vi "ngi data packet JBV.vi"(0 "Dust Data Notifications":T9, 5 "list only event > 0":bool, 9 "mac adresses":T3, 12 "use correction":bool=TRUE) -> (1 "output waveforms":cluster{waveform(dbl)[], waveform(dbl)[]}, 2 "NGI  packets dust":cluster{"MAc Adress":string, "data":string}[](array[cluster]), 3 "Adjustable Parameters":T4(array[cluster]) {"ACMP0 ch" items=["Geophone 1"=0, "Geophone 2"=3, "Geophone 3"=4, "Geophone 4"=5]; "ACMP1 ch" items=["Geophone 2"=1, "Geophone 3"=2, "Geophone 4"=3]}, 6 "Avalanch JBV":T1(array[cluster]) {"A2 mean" format="%.1f"; "A1 mean" format="%.1f"; "A1 std" format="%.1f"; "A2 std" format="%.1f"}, 8 "Recent events":T5(array[cluster]) {"SPS" format="%.1f"}, 10 "Is Logging":T7(array[cluster]), 11 "AUX data":T2(array[cluster]) {"Node configuration"."configuration" items=[""=100, "Radio Repeater"=0, "Geofon"=1, "Sensornode"=2, "Infralyd"=4, "Jernbane"=3]; "Node configuration"."radio config" items=[""=100, "Smartmesh IP"=0]; "batteri (V)" format="%.3g"; "temperatur (c)" format="%.1g"; "?" format="%#.5g"}, 13 "Downloaded dataset":T6(array[cluster]), 14 "last packet type":u8[](array[numeric]), 15 "Avalanch Packets":T8(array[cluster]) {"A1 std" format="%.1g"; "A2 std" format="%.1g"; "A3 std" format="%.1g"; "A4 std" format="%.1g"; "A1 rat" format="%.1g"; "A2 rat" format="%.1g"; "A3 rat" format="%.1g"; "A4 rat" format="%.1g"})   [LabVIEW 2017]
panel:
  out "data":string
  out "sps":dbl
  out "num_samples":u16
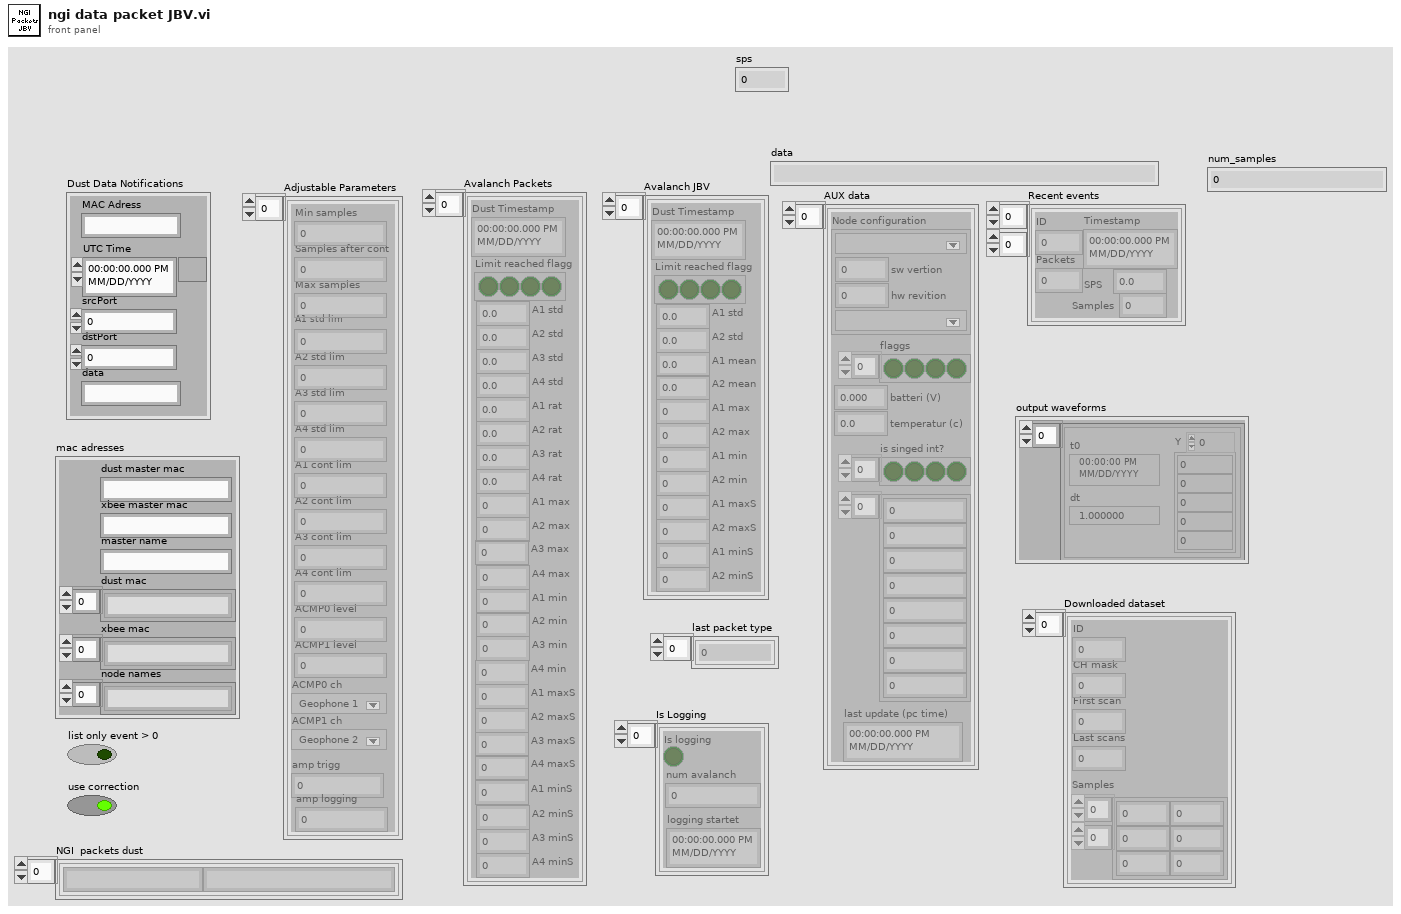
[diagram p1: front panel]
types:
  T1 = cluster{"Dust Timestamp":timestamp, "Limit reached flagg":bool[], "A1 std":sgl, "A2 std":sgl, "A1 mean":sgl, "A2 mean":sgl, "A1 max":i32, "A2 max":i32, "A1 min":i32, "A2 min":i32, "A1 maxS":u16, "A2 maxS":u16, "A1 minS":u16, "A2 minS":u16}[]
  T2 = cluster{"Node configuration":cluster{"configuration":u8, "sw vertion":u8, "hw revition":u8, "radio config":u8}, "flaggs":bool[], "batteri (V)":dbl, "temperatur (c)":dbl, "is singed int?":bool[], dbl[], "last update (pc time)":timestamp}[]
  T3 = cluster{"dust master mac":string, "xbee master mac":string, "master name":string, "dust mac":string[], "xbee mac":string[], "node names":string[]}
  T4 = cluster{"Min samples":u32, "Samples after cont":u32, "Max samples":u32, "A1 std lim":sgl, "A2 std lim":sgl, "A3 std lim":sgl, "A4 std lim":sgl, "A1 cont lim":sgl, "A2 cont lim":sgl, "A3 cont lim":sgl, "A4 cont lim":sgl, "ACMP0 level":u32, "ACMP1 level":u32, "ACMP0 ch":u8, "ACMP1 ch":u8, "amp trigg":u16, "amp logging":u16}[]
  T5 = cluster{"ID":u16, "Timestamp":timestamp, "Packets":u16, "SPS":dbl, "Samples":u16}[][]
  T6 = cluster{"ID":u16, "CH mask":u8, "First scan":u32, "Last scans":u32, "Samples":i32[][]}[]
  T7 = cluster{"Is logging":bool, "num avalanch":u16, "logging startet":timestamp}[]
  T8 = cluster{"Dust Timestamp":timestamp, "Limit reached flagg":bool[], "A1 std":sgl, "A2 std":sgl, "A3 std":sgl, "A4 std":sgl, "A1 rat":sgl, "A2 rat":sgl, "A3 rat":sgl, "A4 rat":sgl, "A1 max":u16, "A2 max":u16, "A3 max":u16, "A4 max":u16, "A1 min":u16, "A2 min":u16, "A3 min":u16, "A4 min":u16, "A1 maxS":u16, "A2 maxS":u16, "A3 maxS":u16, "A4 maxS":u16, "A1 minS":u16, "A2 minS":u16, "A3 minS":u16, "A4 minS":u16}[]
  T9 = cluster{"MAC Adress":string, "UTC Time":timestamp, "srcPort":u16, "dstPort":u16, "data":string}
  T10 = cluster{"Dust Timestamp":timestamp, "Boolean array":bool[], "default value 1":sgl, "default value 1":sgl, "default value 1":sgl, "default value 1":sgl, "default value 1":i32, "default value 1":i32, "default value 1":i32, "default value 1":i32, "default value 1":u16, "default value 1":u16, "default value 1":u16, "default value 1":u16}
  T11 = cluster{cluster{"configuration":i32, "sw vertion":u8, "hw revition":u8, "radio config":i32}, "flaggs":bool[], "batteri (V)":dbl, "temperatur (c)":dbl, "singed int":bool[], dbl[], "last update (pc time)":timestamp}
  T12 = cluster{"Dust Timestamp":timestamp, "Boolean array":bool[], "default value 1":sgl, "default value 1":sgl, "default value 1":sgl, "default value 1":sgl, "default value 1":sgl, "default value 1":sgl, "default value 1":sgl, "default value 1":sgl, "default value 1":u16, "default value 1":u16, "default value 1":u16, "default value 1":u16, "default value 1":u16, "default value 1":u16, "default value 1":u16, "default value 1":u16, "default value 1":u16, "default value 1":u16, "default value 1":u16, "default value 1":u16, "default value 2":u16, "default value 3":u16, "default value 4":u16, "default value 5":u16}
  T13 = cluster{"ID":u16, "Timestamp":timestamp, "Num Packets":u16, "SPS":dbl, "Num samples":u16}
  T14 = cluster{bool, "default value 1":u16, "seconds since 1Jan1904":timestamp}
  T15 = cluster{"default value 1":u16, "default value 1":u8, "default value 1":u32, "default value 1":u32, i32[][]}
  T16 = cluster{"default value 1":u32, "default value 1":u32, "default value 1":u32, "default value 1":sgl, "default value 1":sgl, "default value 1":sgl, "default value 1":sgl, "default value 1":sgl, "default value 1":sgl, "default value 1":sgl, "default value 1":sgl, "default value 1":u32, "default value 1":u32, "default value 1":u8, "default value 1":u8, "default value 2":u16, "default value 3":u16}
  T17 = cluster{"ID":u16, "Timestamp":timestamp, "Num":u16, "Rødt lys":dbl, "Num 2":i32}
  T18 = enum16{"big-endian, network order", "native, host order", "little-endian"}
  T19 = cluster{"Dust Timestamp":timestamp, "Boolean array":bool[], "default value 1":sgl, "default value 1":sgl, "default value 1":sgl, "default value 1":sgl, "default value 1":sgl, "default value 1":sgl, "default value 1":sgl, "default value 1":sgl, "default value 1":u16, "default value 1":u16, "default value 1":u16, "default value 1":u16, "default value 1":u16, "default value 1":u16, "default value 1":u16, "default value 1":u16, "default value 1":u16, "default value 1":u16, "default value 1":u16, "default value 1":u16, "default value 2":u16, "default value 3":u16, "default value 4":u16, "default value 5":u16}[]
  T20 = cluster{cluster{"configuration":i32, "sw vertion":u8, "hw revition":u8, "radio config":i32}, "flaggs":bool[], "batteri (V)":dbl, "temperatur (c)":dbl, "singed int":bool[], dbl[], "last update (pc time)":timestamp}[]
  T21 = cluster{"Dust Timestamp":timestamp, "Boolean array":bool[], "default value 1":sgl, "default value 1":sgl, "default value 1":sgl, "default value 1":sgl, "default value 1":i32, "default value 1":i32, "default value 1":i32, "default value 1":i32, "default value 1":u16, "default value 1":u16, "default value 1":u16, "default value 1":u16}[]
  T22 = cluster{"ID":u16, "Timestamp":timestamp, "Num Packets":u16, "SPS":dbl, "Num samples":u16}[][]
  T23 = cluster{"default value 1":u32, "default value 1":u32, "default value 1":u32, "default value 1":sgl, "default value 1":sgl, "default value 1":sgl, "default value 1":sgl, "default value 1":sgl, "default value 1":sgl, "default value 1":sgl, "default value 1":sgl, "default value 1":u32, "default value 1":u32, "default value 1":u8, "default value 1":u8, "default value 2":u16, "default value 3":u16}[]
  T24 = cluster{bool, "default value 1":u16, "seconds since 1Jan1904":timestamp}[]
  T25 = cluster{"default value 1":u16, "default value 1":u8, "default value 1":u32, "default value 1":u32, i32[][]}[]
  T26 = cluster{"Dust Timestamp":timestamp, "Boolean array":bool[], "default value 1":sgl, "default value 1":sgl, "default value 1":sgl, "default value 1":sgl, sgl, sgl, sgl, sgl, "default value 1":u16, "default value 1":u16, "default value 1":u16, "default value 1":u16, "default value 1":u16, "default value 1":u16, "default value 1":u16, "default value 1":u16, "default value 1":u16, "default value 1":u16, "default value 1":u16, "default value 1":u16, "default value 1":u16, "default value 1":u16, "default value 1":u16, "default value 1":u16}
  T27 = cluster{"Dust Timestamp":timestamp, "Boolean array":bool[], "default value 1":sgl, "default value 1":sgl, "default value 1":sgl, "default value 1":sgl, i32, i32, i32, i32, "default value 1":u16, "default value 1":u16, "default value 1":u16, "default value 1":u16}
  T28 = cluster{"Dust Timestamp":timestamp, "Boolean array":bool[], "default value 1":sgl, "default value 1":sgl, "default value 1":sgl, "default value 1":sgl, i32, "default value 1":i32, i32, "default value 1":i32, "default value 1":u16, "default value 1":u16, "default value 1":u16, "default value 1":u16}
  T29 = cluster{"default value 1":u16, "Dust Timestamp":timestamp, "default value 1":u16, dbl, "default value 1":u16}
  T30 = cluster{"ID":u16, "Timestamp":timestamp, "Num Packets":u16, "SPS":dbl, "Num 2":i32}[]
  T31 = cluster{"default value 1":u32, "default value 1":u32, "default value 1":u32, "default value 1":sgl, "default value 1":sgl, "default value 1":sgl, "default value 1":sgl, "default value 1":sgl, "default value 1":sgl, "default value 1":sgl, "default value 1":sgl, u32, u32, "default value 1":u8, "default value 1":u8, "default value 1":u16, "default value 1":u16}
  T32 = cluster{cluster{u8, u8, u8, u8}, "Boolean array":bool[], dbl, dbl, "Boolean array":bool[], dbl[], "seconds since 1Jan1904":timestamp}
  T33 = cluster{"ID":u16, "Timestamp":timestamp, "Num Packets":u16, "SPS":dbl, "Num 2":i32}[][]
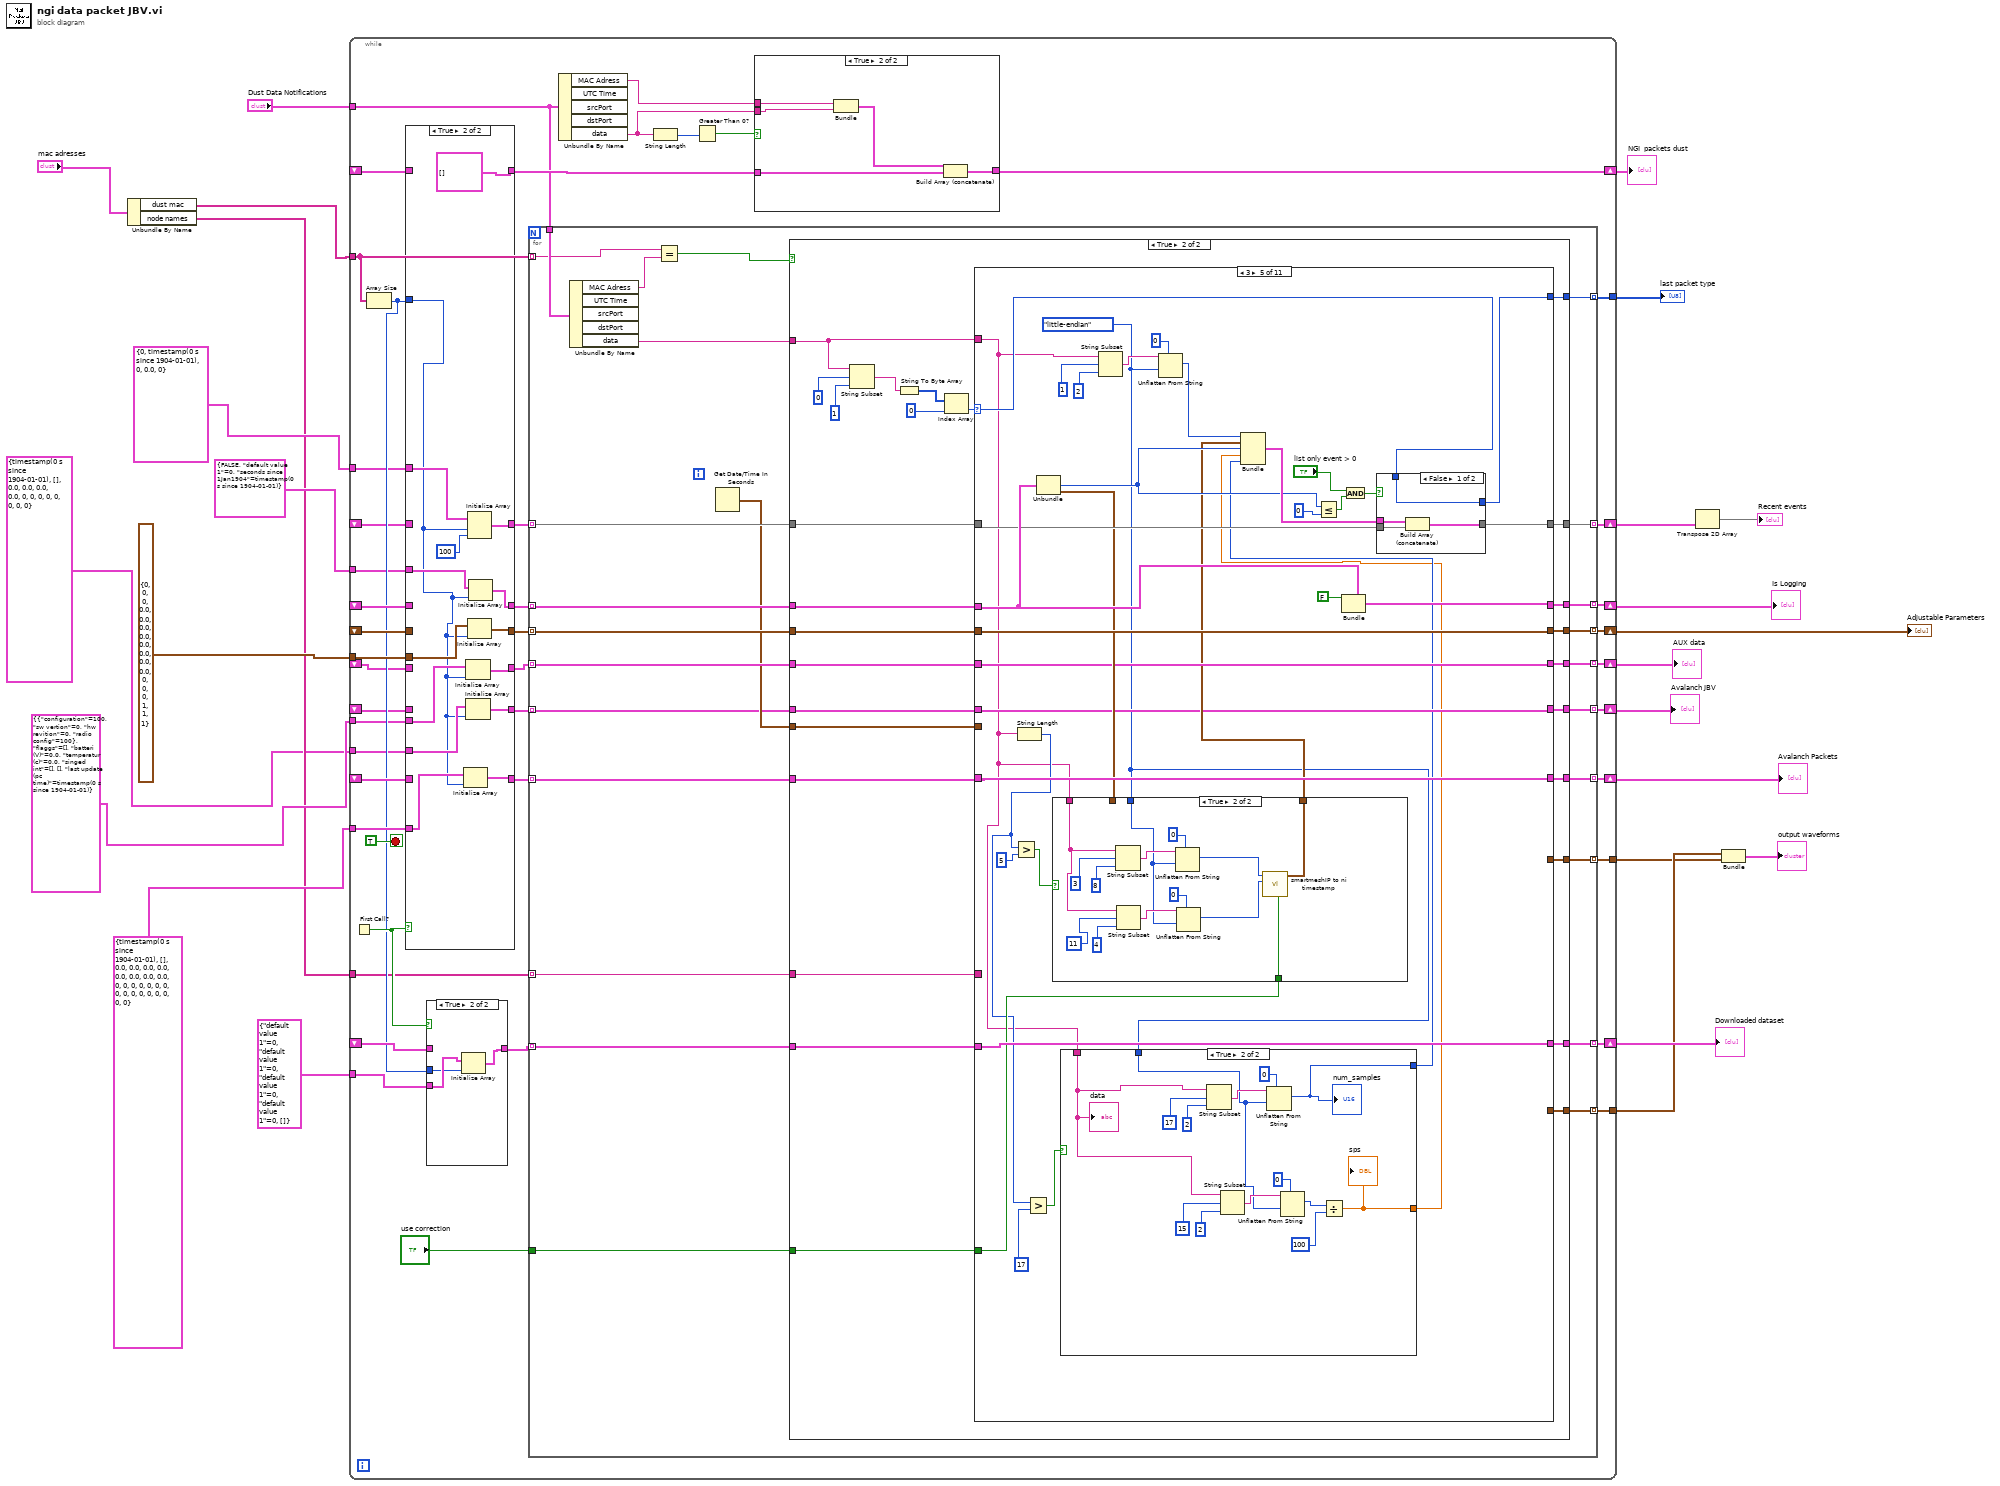
[diagram p0: block diagram]
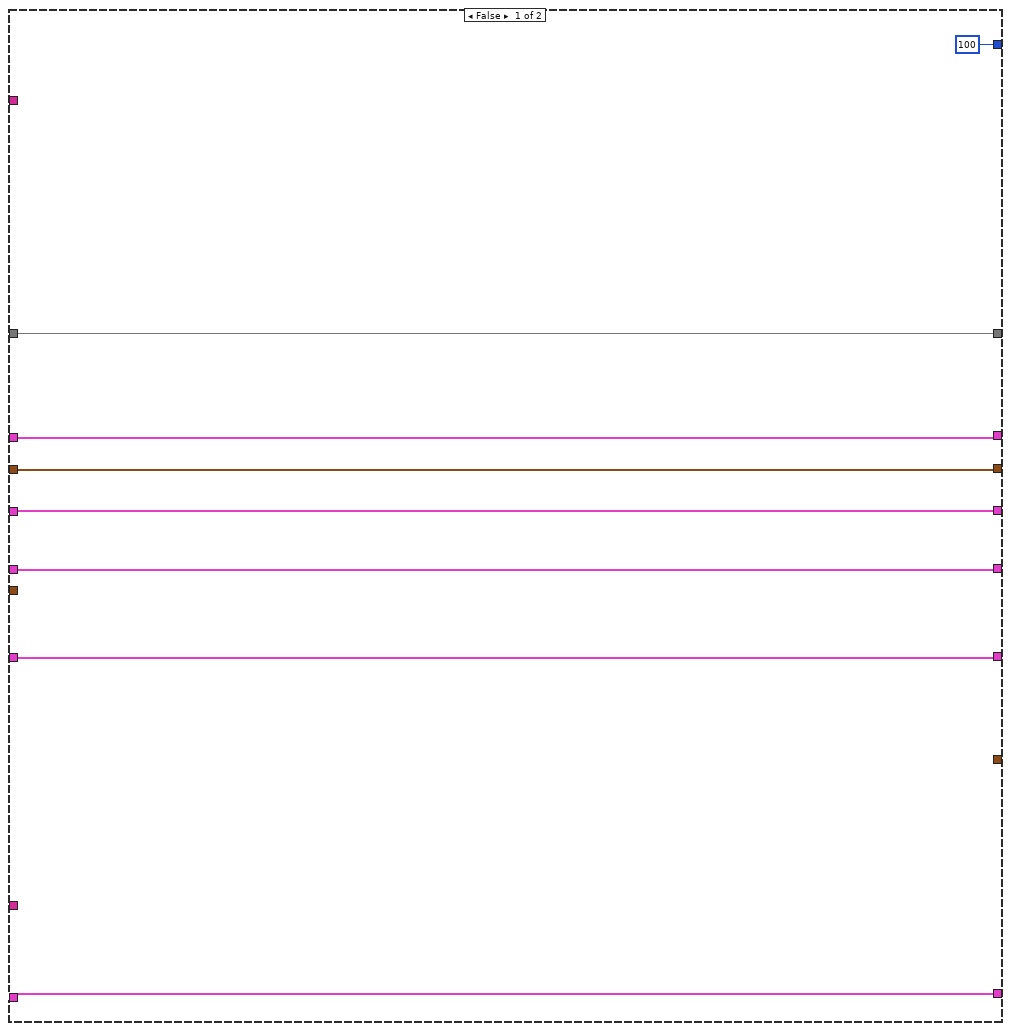
[diagram p3: hidden frame]
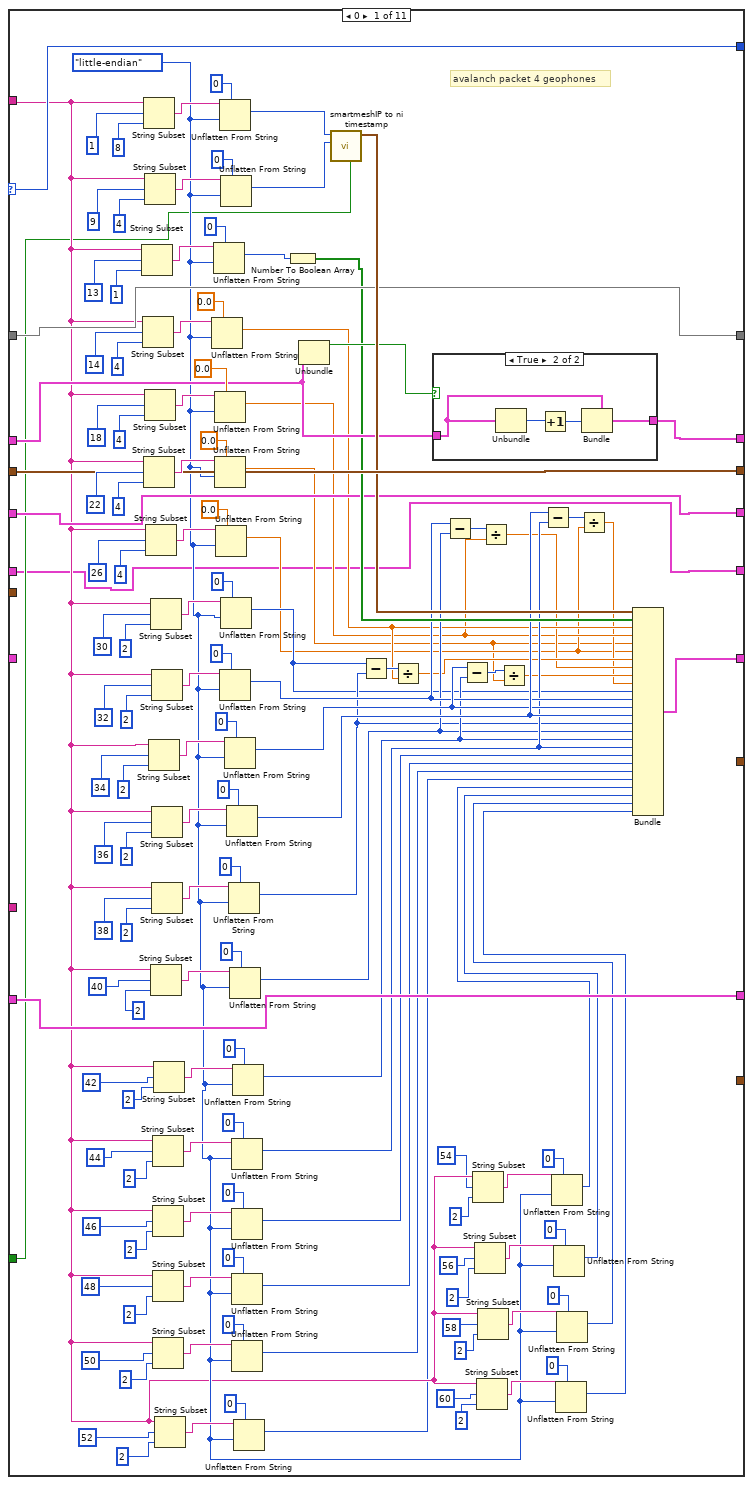
[diagram p4: hidden frame]
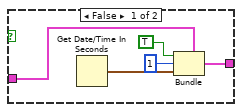
[diagram p5: hidden frame]
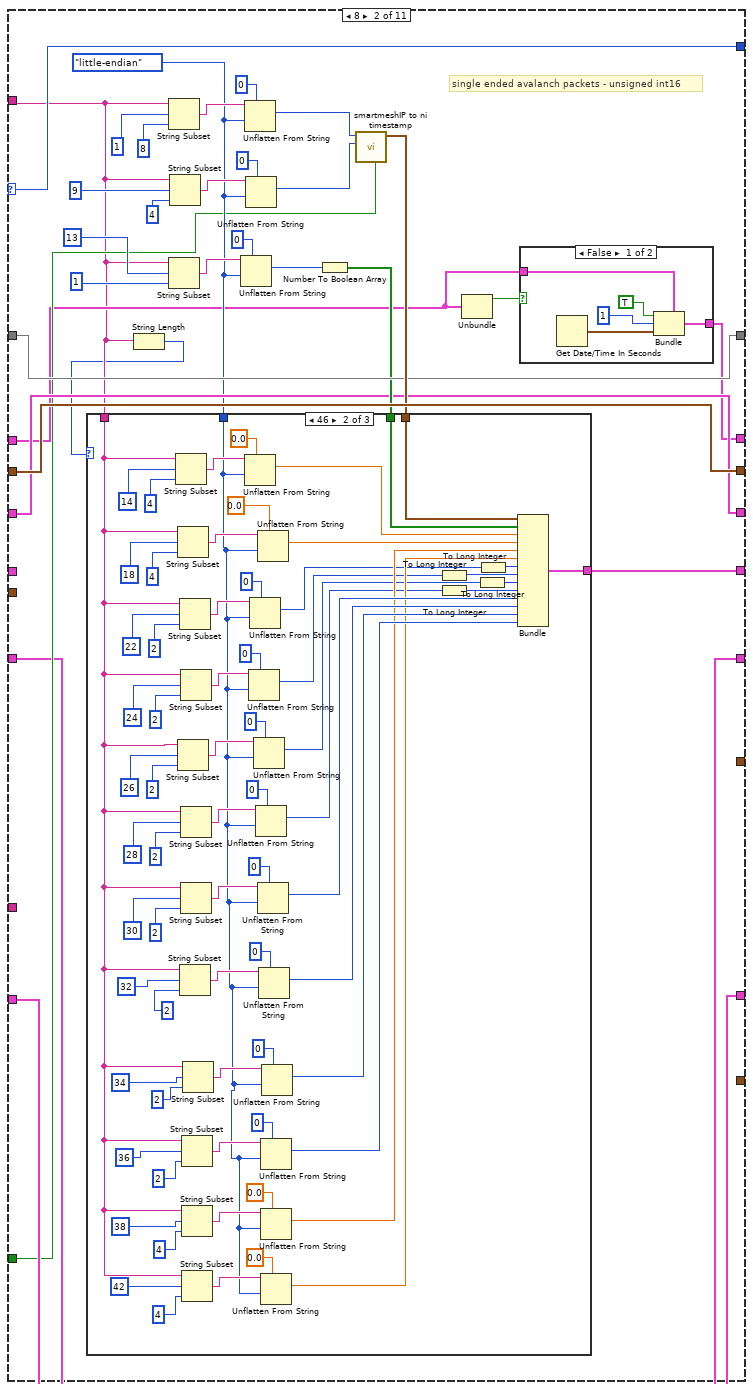
[diagram p6: hidden frame]
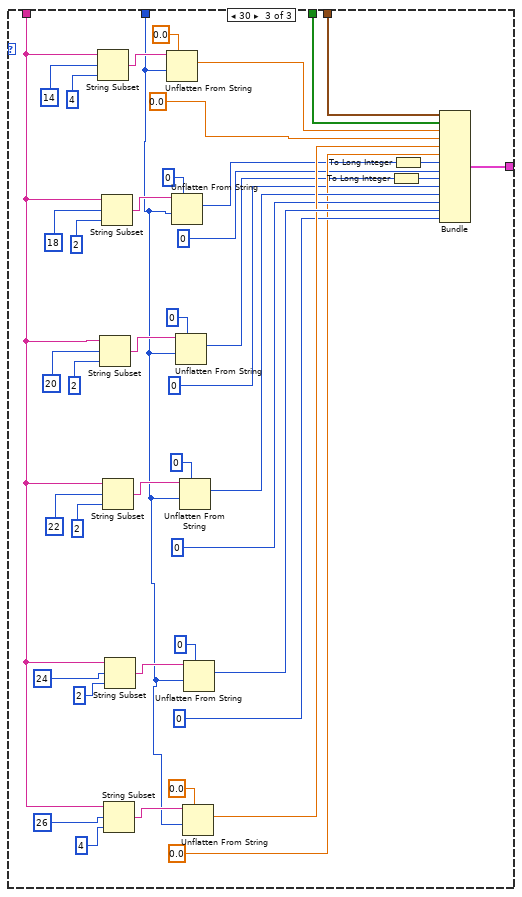
[diagram p8: hidden frame]
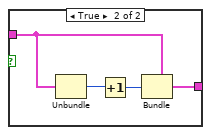
[diagram p9: hidden frame]
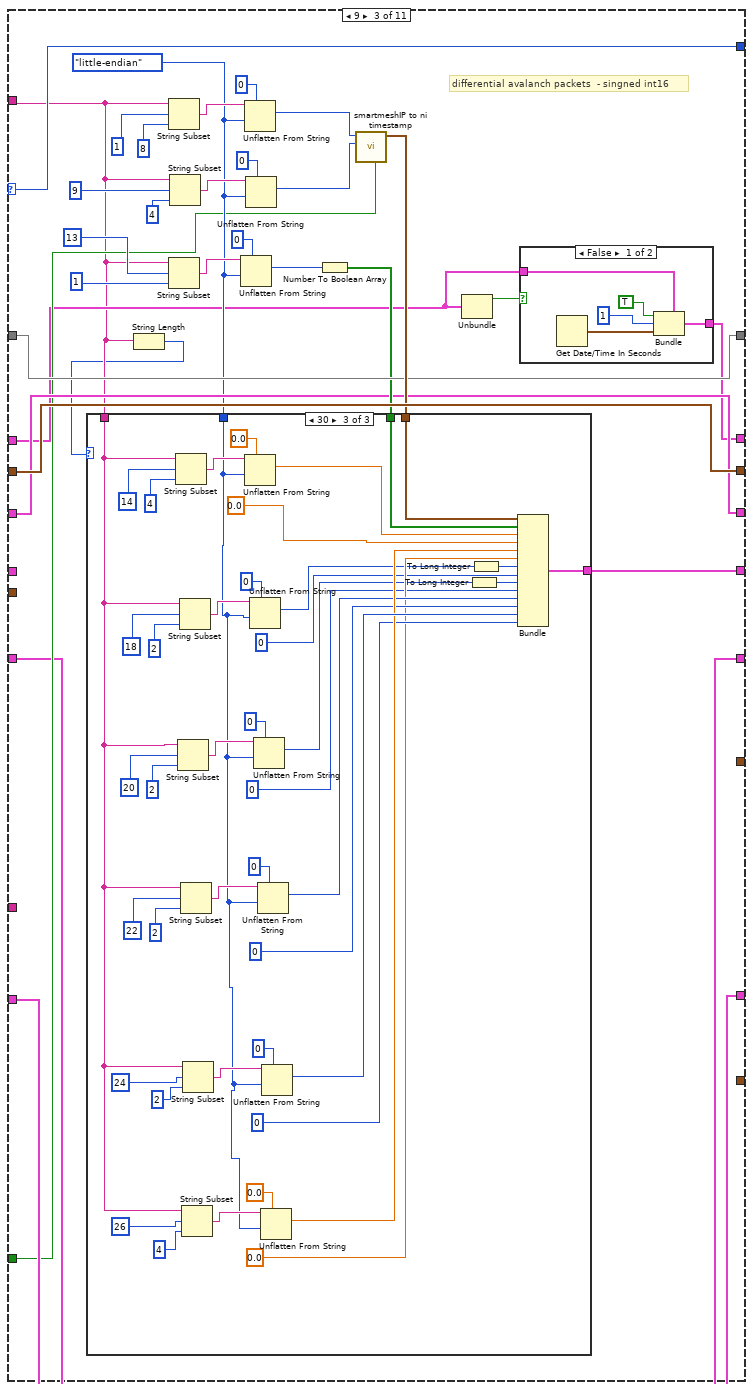
[diagram p10: hidden frame]
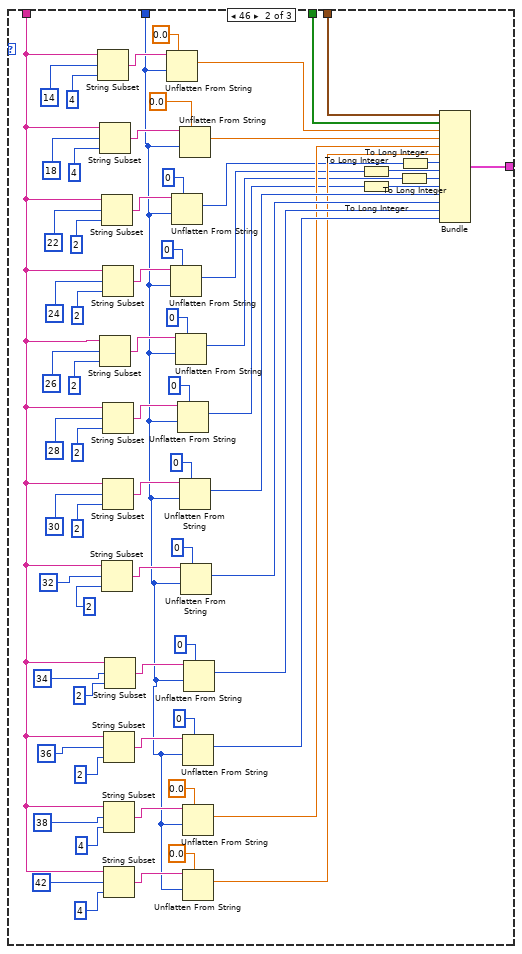
[diagram p12: hidden frame]
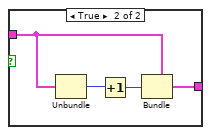
[diagram p13: hidden frame]
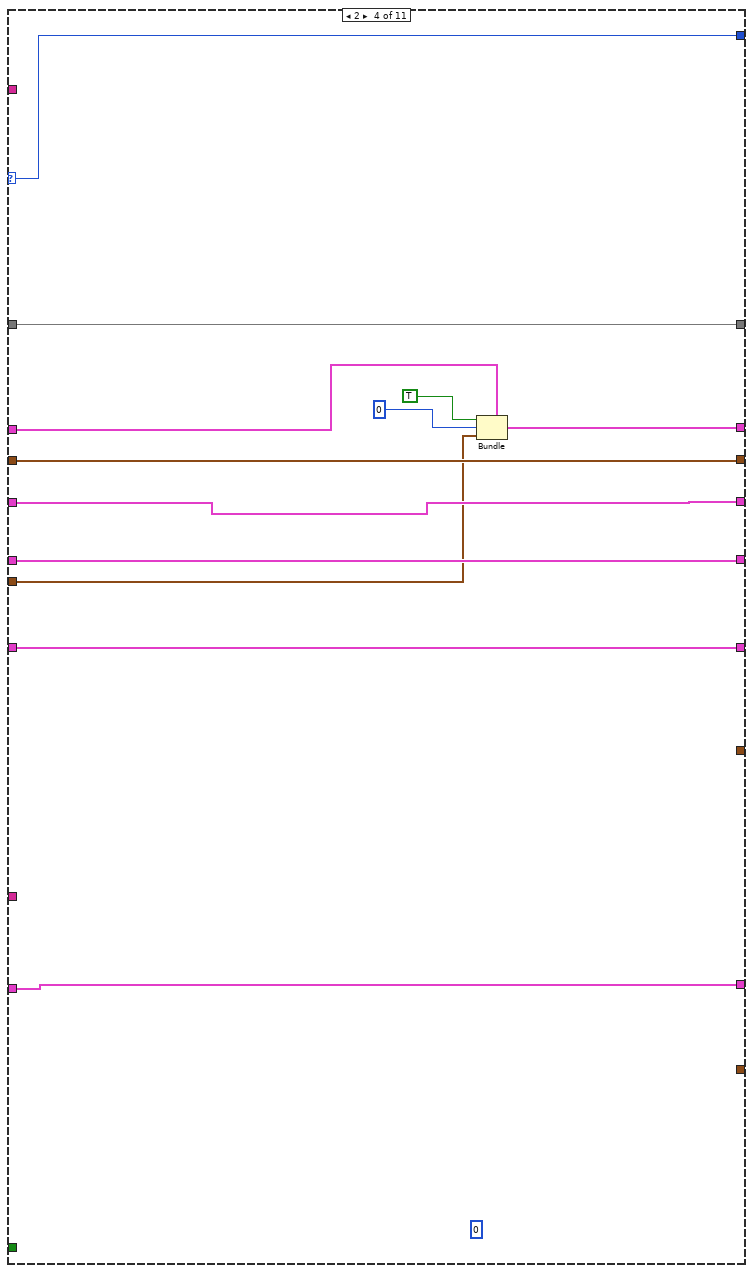
[diagram p14: hidden frame]
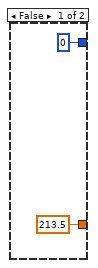
[diagram p15: hidden frame]
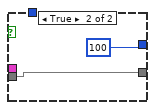
[diagram p16: hidden frame]
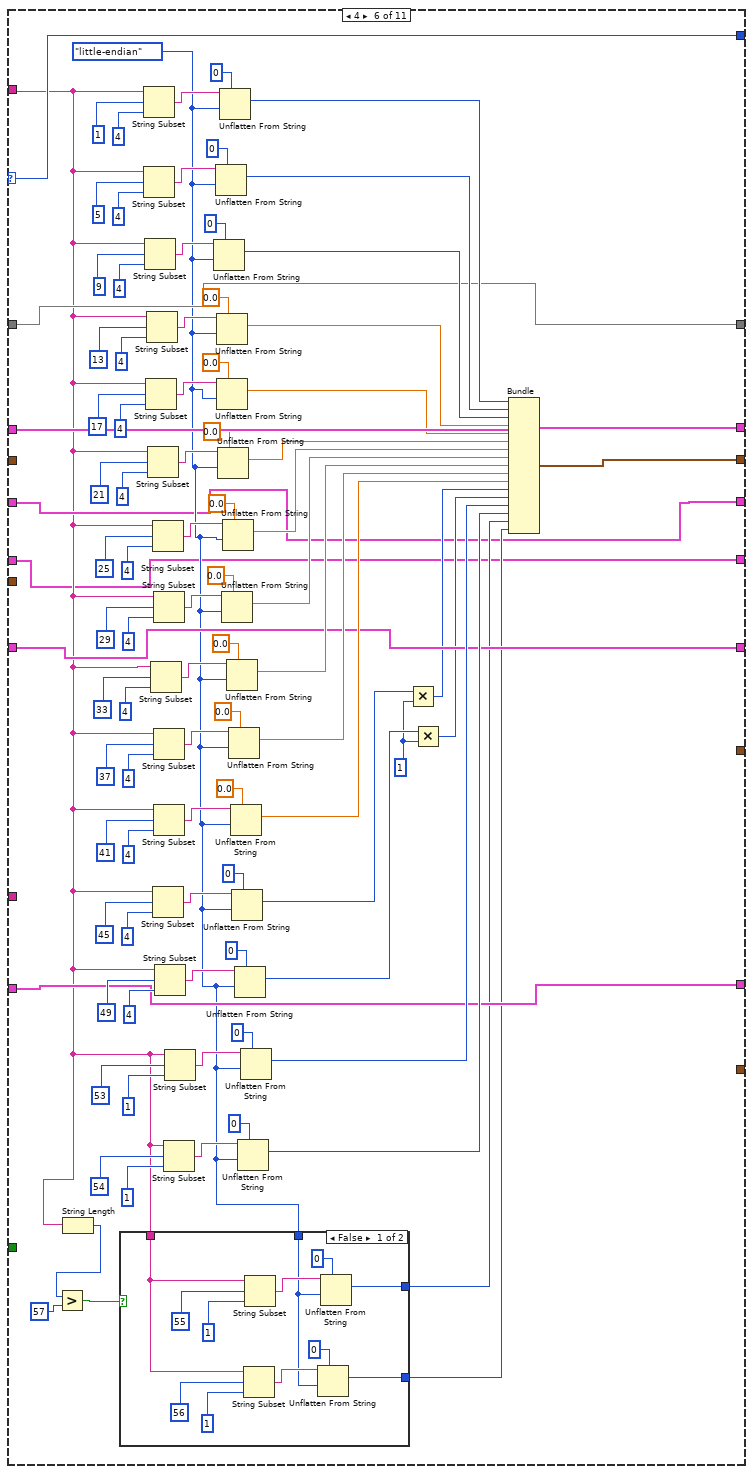
[diagram p18: hidden frame]
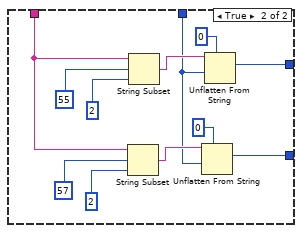
[diagram p19: hidden frame]
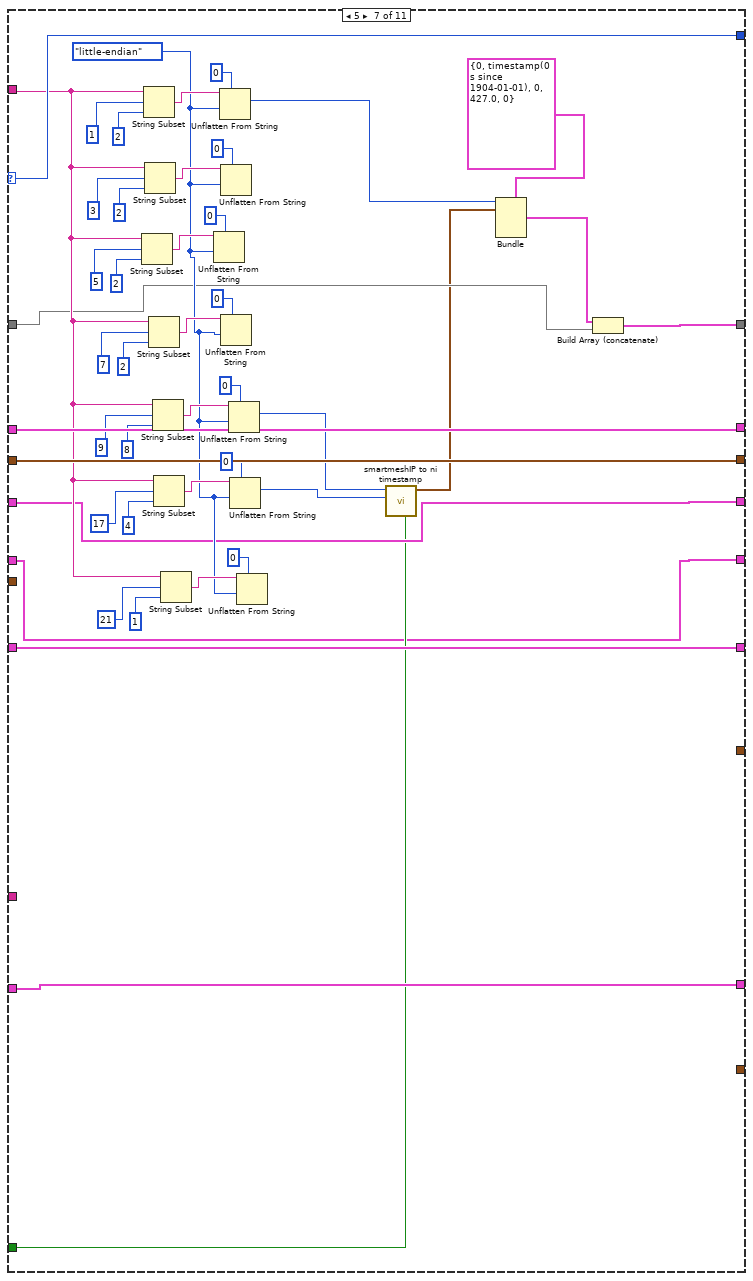
[diagram p20: hidden frame]
diagram:
  n1 = Unbundle By Name("mac adresses") -> ("dust mac"=w11:string[], "node names"=w3:string[])
  n2 = while {
    tunnel: "Dust Data Notifications" -> [w61]
    tunnel: w11 -> [w60]
    shift-right: [w64] -> w23
    shift-left: _ -> [w62]
    shift-right: [w59] -> w17
    shift-left: _ -> [w57]
    shift-right: [w56] -> w12
    shift-left: _ -> [w55]
    tunnel: T16 {"default value 1"=0, "default value 1"=0, "default value 1"=0, "default value 1"=0.0, "default value 1"=0.0, "default value 1"=0.0, "default value 1"=0.0, "default value 1"=0.0, "default value 1"=0.0, "default value 1"=0.0, "default value 1"=0.0, "default value 1"=0, "default value 1"=0, "default value 1"=0, "default value 1"=1, "default value 2"=1, "default value 3"=1} -> [w53]
    tunnel: [w52] -> w21
    shift-right: [w51] -> w19
    shift-left: _ -> [w49]
    tunnel: T12 {"Dust Timestamp"=timestamp(0 s since 1904-01-01), "Boolean array"=[], "default value 1"=0.0, "default value 1"=0.0, "default value 1"=0.0, "default value 1"=0.0, "default value 1"=0.0, "default value 1"=0.0, "default value 1"=0.0, "default value 1"=0.0, "default value 1"=0, "default value 1"=0, "default value 1"=0, "default value 1"=0, "default value 1"=0, "default value 1"=0, "default value 1"=0, "default value 1"=0, "default value 1"=0, "default value 1"=0, "default value 1"=0, "default value 1"=0, "default value 2"=0, "default value 3"=0, "default value 4"=0, "default value 5"=0} -> [w48]
    shift-right: [w47] -> w16
    shift-left: _ -> [w45]
    tunnel: T15 {"default value 1"=0, "default value 1"=0, "default value 1"=0, "default value 1"=0, []} -> [w44]
    shift-right: [w38] -> w14
    shift-left: _ -> [w37]
    tunnel: T14 {FALSE, "default value 1"=0, "seconds since 1Jan1904"=timestamp(0 s since 1904-01-01)} -> [w40]
    tunnel: T13 {"ID"=0, "Timestamp"=timestamp(0 s since 1904-01-01), "Num Packets"=0, "SPS"=0.0, "Num samples"=0} -> [w39]
    tunnel: [w36] -> w5
    tunnel: w3 -> [w35]
    tunnel: [w34] -> w6
    shift-right: [w33] -> w8
    shift-left: _ -> [w31]
    tunnel: T11 {{"configuration"=100, "sw vertion"=0, "hw revition"=0, "radio config"=100}, "flaggs"=[], "batteri (V)"=0.0, "temperatur (c)"=0.0, "singed int"=[], [], "last update (pc time)"=timestamp(0 s since 1904-01-01)} -> [w30]
    shift-right: [w28] -> w2
    shift-left: _ -> [w27]
    tunnel: T10 {"Dust Timestamp"=timestamp(0 s since 1904-01-01), "Boolean array"=[], "default value 1"=0.0, "default value 1"=0.0, "default value 1"=0.0, "default value 1"=0.0, "default value 1"=0, "default value 1"=0, "default value 1"=0, "default value 1"=0, "default value 1"=0, "default value 1"=0, "default value 1"=0, "default value 1"=0} -> [w25]
    stop <- TRUE stop-if-true
    n3 = First Call?() -> (First Call?: T/F=w42:bool)
    n4 = Array Size(array=w60) -> (size(s)=w41:i32)
    n5 = case shown="True" w42 {
      tunnel: [w1077 cluster{"MAc Adress":string, "data":string}[] []] -> w63
      tunnel: w62 -> [w1077 _]
      tunnel: w41 -> [_ w1079]
      tunnel: [w1076 w1085] -> w58
      tunnel: w57 -> [w1076 _]
      tunnel: [w1075 w1091] -> w54
      tunnel: w55 -> [w1075 _]
      tunnel: w53 -> [_ w1092]
      tunnel: [w1074 w1090] -> w50
      tunnel: w49 -> [w1074 _]
      tunnel: w48 -> [_ w1089]
      tunnel: [w1073 w1083] -> w43
      tunnel: w37 -> [w1073 _]
      tunnel: w40 -> [_ w1086]
      tunnel: w39 -> [_ w1084]
      tunnel: [w1072 w1081] -> w32
      tunnel: w31 -> [w1072 _]
      tunnel: w30 -> [_ w1082]
      tunnel: w27 -> [w1071 _]
      tunnel: [w1071 w1078] -> w26
      tunnel: w25 -> [_ w1080]
      frame False {
      }
      frame True {
        n6 = Initialize Array(w1089, w1079) -> (w1090:T19)
        n7 = Initialize Array(w1082, w1079) -> (w1081:T20)
        n8 = Initialize Array(w1080, w1079) -> (w1078:T21)
        n9 = Initialize Array(w1084, w1079, 100 ("dimension size")) -> (w1083:T22)
        n10 = Initialize Array(w1092, w1079) -> (w1091:T23)
        n11 = Initialize Array(w1086, w1079) -> (w1085:T24)
      }
    }
    n12 = case shown="True" w42 {
      tunnel: [w70 w71] -> w46
      tunnel: w45 -> [w70 _]
      tunnel: w44 -> [_ w73]
      tunnel: w41 -> [_ w72]
      frame False {
      }
      frame True {
        n13 = Initialize Array(w73, w72) -> (w71:T25)
      }
    }
    n14 = for {
      tunnel: w60 -> [w97] mode=indexing
      tunnel: w61 -> [w98]
      tunnel: [w96] -> w59 mode=indexing
      tunnel: w58 -> [w95] mode=indexing
      tunnel: [w94] -> w56 mode=indexing
      tunnel: w54 -> [w93] mode=indexing
      tunnel: [w92] -> w52 mode=indexing
      tunnel: [w91] -> w51 mode=indexing
      tunnel: w50 -> [w90] mode=indexing
      tunnel: [w89] -> w47 mode=indexing
      tunnel: w46 -> [w88] mode=indexing
      tunnel: [w87] -> w38 mode=indexing
      tunnel: w43 -> [w86] mode=indexing
      tunnel: [w85] -> w36 mode=indexing
      tunnel: w35 -> [w84] mode=indexing
      tunnel: [w83] -> w34 mode=indexing
      tunnel: [w82] -> w33 mode=indexing
      tunnel: w32 -> [w81] mode=indexing
      tunnel: "use correction" -> [w79]
      tunnel: [w75] -> w28 mode=indexing
      tunnel: w26 -> [w74] mode=indexing
      n15 = Unbundle By Name(w98) -> ("MAC Adress"=w80:string, "data"=w76:string)  [unwired: 3 out]
      n16 = Equal?(x=w97, y=w80) -> (x = y?=w77:bool)
      n17 = Get Date/Time In Seconds() -> (seconds since 1Jan1904=w78:timestamp)
      n18 = case shown="True" w77 {
        tunnel: w76 -> [_ w121]
        tunnel: [w106 w132] -> w96
        tunnel: w95 -> [w106 w133]
        tunnel: [w105 w131] -> w94
        tunnel: w93 -> [w105 w130]
        tunnel: [u8 100 w129] -> w92
        tunnel: [w104 w128] -> w91
        tunnel: w90 -> [w104 w127]
        tunnel: [w103 w119] -> w89
        tunnel: w88 -> [w103 w118]
        tunnel: w78 -> [_ w117]
        tunnel: [w102 w116] -> w87
        tunnel: w86 -> [w102 w115]
        tunnel: [_ w114] -> w85
        tunnel: w84 -> [_ w113]
        tunnel: [_ w112] -> w83
        tunnel: [w100 w111] -> w82
        tunnel: w81 -> [w100 w110]
        tunnel: w79 -> [_ w109]
        tunnel: [w99 w108] -> w75
        tunnel: w74 -> [w99 w107]
        frame False {
        }
        frame True {
          n19 = String Subset(string=w121, offset (0)=0, length (rest)=1 ("length (rest)")) -> (substring=w126:string)
          n20 = String To Byte Array(string=w126) -> (unsigned byte array=w125:u8[])
          n21 = Index Array(array=w125, index=0) -> (element=w120:u8)
          n22 = case shown="3" w120 {
            selector: w120 -> [w226 w303 w455 w595 w611 w686 w823 w864 w920 w1015 _]
            tunnel: w133 -> [w210 w285 w437 w591 w621 w758 w817 w857 w913 w1009 w1070]
            tunnel: [w209 w283 w435 w590 w623 w758 w817 w857 w913 w1009 w1070] -> w132
            tunnel: w121 -> [w174 w282 w434 _ w597 w673 w800 w846 w902 w948 _]
            tunnel: [w225 w302 w454 w596 w631 w730 w818 w858 w914 w1010 w1069] -> w131
            tunnel: w130 -> [w225 w302 w454 w596 w631 _ w818 w858 w914 w1010 w1069]
            tunnel: [w226 w303 w455 w595 w610 w686 w823 w864 w920 w1015 u8 100] -> w129
            tunnel: [w223 w287 w439 w594 w630 w685 w816 w856 w912 w1008 w1068] -> w128
            tunnel: w127 -> [_ w287 w439 w594 w630 w685 w816 w856 w912 w1008 w1068]
            tunnel: [w216 w297 w449 w593 w629 w684 w797 w842 w898 w1007 w1067] -> w119
            tunnel: w118 -> [w216 w297 w449 w593 w629 w684 w797 _ _ w1007 w1067]
            tunnel: w117 -> [_ _ _ w585 _ _ _ _ _ w954 _]
            tunnel: [w212 w293 w445 w592 w624 w683 w793 w843 w899 w1006 w1066] -> w116
            tunnel: w115 -> [w212 w293 w445 w592 w620 w683 w794 w843 w899 w1006 w1066]
            tunnel: [_ _ _ _ _ _ _ _ _ w1002 _] -> w114
            tunnel: w113 -> [_ _ _ _ _ _ _ _ _ w996 _]
            tunnel: [_ _ _ _ _ _ _ _ _ w995 _] -> w112
            tunnel: [w206 w290 w442 w587 w615 w674 w788 w840 w896 w975 w1064] -> w111
            tunnel: w110 -> [w206 w290 w442 w587 w615 w674 w788 w840 w896 _ w1064]
            tunnel: w109 -> [w135 w288 w440 _ w604 _ w787 _ _ _ _]
            tunnel: [w134 w286 w438 w586 w605 w669 w786 w832 w888 w944 w1063] -> w108
            tunnel: w107 -> [w134 _ _ w586 w605 w669 w786 w832 w888 w944 w1063]
            frame 0 {
              w185 = T18."little-endian" ("byte order (0:big-endian, network order)")
              # "avalanch packet 4 geophones"
              n23 = String Subset(string=w174, offset (0)=13, length (rest)=1 ("length (rest)")) -> (substring=w236:string)
              n24 = String Subset(string=w174, offset (0)=14, length (rest)=4 ("length (rest)")) -> (substring=w235:string)
              n25 = String Subset(string=w174, offset (0)=1, length (rest)=8 ("length (rest)")) -> (substring=w249:string)
              n26 = String Subset(string=w174, offset (0)=22, length (rest)=4 ("length (rest)")) -> (substring=w233:string)
              n27 = String Subset(string=w174, offset (0)=9, length (rest)=4 ("length (rest)")) -> (substring=w219:string)
              n28 = String Subset(string=w174, offset (0)=18, length (rest)=4 ("length (rest)")) -> (substring=w234:string)
              n29 = String Subset(string=w174, offset (0)=26, length (rest)=4 ("length (rest)")) -> (substring=w232:string)
              n30 = String Subset(string=w174, offset (0)=34, length (rest)=2 ("length (rest)")) -> (substring=w229:string)
              n31 = String Subset(string=w174, offset (0)=30, length (rest)=2 ("length (rest)")) -> (substring=w231:string)
              n32 = String Subset(string=w174, offset (0)=40, length (rest)=2 ("length (rest)")) -> (substring=w222:string)
              n33 = String Subset(string=w174, offset (0)=32, length (rest)=2 ("length (rest)")) -> (substring=w230:string)
              n34 = String Subset(string=w174, offset (0)=36, length (rest)=2 ("length (rest)")) -> (substring=w228:string)
              n35 = String Subset(string=w174, offset (0)=38, length (rest)=2 ("length (rest)")) -> (substring=w227:string)
              n36 = String Subset(string=w174, offset (0)=44, length (rest)=2 ("length (rest)")) -> (substring=w202:string)
              n37 = String Subset(string=w174, offset (0)=46, length (rest)=2 ("length (rest)")) -> (substring=w200:string)
              n38 = String Subset(string=w174, offset (0)=48, length (rest)=2 ("length (rest)")) -> (substring=w198:string)
              n39 = String Subset(string=w174, offset (0)=50, length (rest)=2 ("length (rest)")) -> (substring=w196:string)
              n40 = String Subset(string=w174, offset (0)=42, length (rest)=2 ("length (rest)")) -> (substring=w204:string)
              n41 = String Subset(string=w174, offset (0)=52, length (rest)=2 ("length (rest)")) -> (substring=w186:string)
              n42 = Unflatten From String(type=sgl 0.0 ("default value 1"), binary string=w235, byte order (0:big-endian, network order)=w185) -> (value=w145:sgl)  [unwired: 2 in, 2 out]
              n43 = Unflatten From String(type=u8 0 ("default value 1"), binary string=w236, byte order (0:big-endian, network order)=w185) -> (value=w208:u8)  [unwired: 2 in, 2 out]
              n44 = Unflatten From String(type=sgl 0.0 ("default value 1"), binary string=w234, byte order (0:big-endian, network order)=w185) -> (value=w142:sgl)  [unwired: 2 in, 2 out]
              n45 = Unflatten From String(type=sgl 0.0 ("default value 1"), binary string=w233, byte order (0:big-endian, network order)=w185) -> (value=w136:sgl)  [unwired: 2 in, 2 out]
              n46 = Unflatten From String(type=sgl 0.0 ("default value 1"), binary string=w232, byte order (0:big-endian, network order)=w185) -> (value=w137:sgl)  [unwired: 2 in, 2 out]
              n47 = Unflatten From String(type=i64 0 ("default value 1"), binary string=w249, byte order (0:big-endian, network order)=w185) -> (value=w215:i64)  [unwired: 2 in, 2 out]
              n48 = Unflatten From String(type=u16 0 ("default value 1"), binary string=w230, byte order (0:big-endian, network order)=w185) -> (value=w153:u16)  [unwired: 2 in, 2 out]
              n49 = Unflatten From String(type=0 ("default value 1"), binary string=w219, byte order (0:big-endian, network order)=w185) -> (value=w214:i32)  [unwired: 2 in, 2 out]
              n50 = Unflatten From String(type=u16 0 ("default value 1"), binary string=w231, byte order (0:big-endian, network order)=w185) -> (value=w147:u16)  [unwired: 2 in, 2 out]
              n51 = Unflatten From String(type=u16 0 ("default value 1"), binary string=w229, byte order (0:big-endian, network order)=w185) -> (value=w154:u16)  [unwired: 2 in, 2 out]
              n52 = Unflatten From String(type=u16 0 ("default value 1"), binary string=w228, byte order (0:big-endian, network order)=w185) -> (value=w155:u16)  [unwired: 2 in, 2 out]
              n53 = Unflatten From String(type=u16 0 ("default value 1"), binary string=w227, byte order (0:big-endian, network order)=w185) -> (value=w149:u16)  [unwired: 2 in, 2 out]
              n54 = Unflatten From String(type=u16 0 ("default value 1"), binary string=w222, byte order (0:big-endian, network order)=w185) -> (value=w150:u16)  [unwired: 2 in, 2 out]
              n55 = Unflatten From String(type=u16 0 ("default value 1"), binary string=w202, byte order (0:big-endian, network order)=w185) -> (value=w152:u16)  [unwired: 2 in, 2 out]
              n56 = Unflatten From String(type=u16 0 ("default value 1"), binary string=w200, byte order (0:big-endian, network order)=w185) -> (value=w156:u16)  [unwired: 2 in, 2 out]
              n57 = Unflatten From String(type=u16 0 ("default value 1"), binary string=w198, byte order (0:big-endian, network order)=w185) -> (value=w157:u16)  [unwired: 2 in, 2 out]
              n58 = Unflatten From String(type=u16 0 ("default value 1"), binary string=w196, byte order (0:big-endian, network order)=w185) -> (value=w158:u16)  [unwired: 2 in, 2 out]
              n59 = Unflatten From String(type=u16 0 ("default value 1"), binary string=w204, byte order (0:big-endian, network order)=w185) -> (value=w151:u16)  [unwired: 2 in, 2 out]
              n60 = Unflatten From String(type=u16 0 ("default value 1"), binary string=w186, byte order (0:big-endian, network order)=w185) -> (value=w159:u16)  [unwired: 2 in, 2 out]
              n61 = Number To Boolean Array(number=w208) -> (Boolean array=w207:bool[])
              n62 = Unbundle(w210) -> (w211:bool)  [unwired: 2 out]
              n63 = call "smartmeshIP to ni timestamp.vi"("use correction"=w135, "microeconds"=w214, "seconds"=w215) -> ("Dust Timestamp"=w213:timestamp)  [unwired: 8 in]
              n64 = Subtract(x=w147, y=w149) -> (x-y=w148:u16)
              n65 = Divide(x=w148, y=w145) -> (x/y=w146:sgl)
              n66 = case shown="True" w211 {
                tunnel: w210 -> [w276 w280]
                tunnel: [w273 w277] -> w209
                frame False {
                  n67 = Get Date/Time In Seconds() -> (seconds since 1Jan1904=w272:timestamp)
                  n68 = Bundle(cluster=w276, TRUE, "default value 1"=u16 1, "seconds since 1Jan1904"=w272) -> (w273:T14)
                }
                frame True {
                  n69 = Unbundle(w280) -> ("default value 1"=w278:u16)  [unwired: 2 out]
                  n70 = Increment(x=w278) -> (x+1=w279:u16)
                  n71 = Bundle(cluster=w280, "default value 1"=w279) -> (w277:T14)  [unwired: 2 in]
                }
              }
              n72 = Subtract(x=w153, y=w150) -> (x-y=w144:u16)
              n73 = Subtract(x=w154, y=w151) -> (x-y=w141:u16)
              n74 = String Subset(string=w174, offset (0)=54, length (rest)=2 ("length (rest)")) -> (substring=w194:string)
              n75 = String Subset(string=w174, offset (0)=56, length (rest)=2 ("length (rest)")) -> (substring=w192:string)
              n76 = String Subset(string=w174, offset (0)=60, length (rest)=2 ("length (rest)")) -> (substring=w188:string)
              n77 = String Subset(string=w174, offset (0)=58, length (rest)=2 ("length (rest)")) -> (substring=w190:string)
              n78 = Divide(x=w144, y=w142) -> (x/y=w143:sgl)
              n79 = Divide(x=w141, y=w136) -> (x/y=w140:sgl)
              n80 = Subtract(x=w155, y=w152) -> (x-y=w139:u16)
              n81 = Unflatten From String(type=u16 0 ("default value 1"), binary string=w194, byte order (0:big-endian, network order)=w185) -> (value=w160:u16)  [unwired: 2 in, 2 out]
              n82 = Unflatten From String(type=u16 0 ("default value 1"), binary string=w192, byte order (0:big-endian, network order)=w185) -> (value=w161:u16)  [unwired: 2 in, 2 out]
              n83 = Unflatten From String(type=u16 0 ("default value 1"), binary string=w188, byte order (0:big-endian, network order)=w185) -> (value=w163:u16)  [unwired: 2 in, 2 out]
              n84 = Unflatten From String(type=u16 0 ("default value 1"), binary string=w190, byte order (0:big-endian, network order)=w185) -> (value=w162:u16)  [unwired: 2 in, 2 out]
              n85 = Divide(x=w139, y=w137) -> (x/y=w138:sgl)
              n86 = Bundle("Dust Timestamp"=w213, "Boolean array"=w207, "default value 1"=w145, "default value 1"=w142, "default value 1"=w136, "default value 1"=w137, w146, w143, w140, w138, "default value 1"=w147, "default value 1"=w153, "default value 1"=w154, "default value 1"=w155, "default value 1"=w149, "default value 1"=w150, "default value 1"=w151, "default value 1"=w152, "default value 1"=w156, "default value 1"=w157, "default value 1"=w158, "default value 1"=w159, "default value 1"=w160, "default value 1"=w161, "default value 1"=w162, "default value 1"=w163) -> (w223:T26)  [unwired: 1 in]
            }
            frame 8 {
              w289 = T18."little-endian" ("byte order (0:big-endian, network order)")
              # "single ended avalanch packets - unsigned int16"
              n87 = String Length(string=w282) -> (length=w281:i32)
              n88 = String Subset(string=w282, offset (0)=1, length (rest)=8 ("length (rest)")) -> (substring=w307:string)
              n89 = String Subset(string=w282, offset (0)=13, length (rest)=1 ("length (rest)")) -> (substring=w304:string)
              n90 = String Subset(string=w282, offset (0)=9, length (rest)=4 ("length (rest)")) -> (substring=w299:string)
              n91 = Unflatten From String(type=u8 0 ("default value 1"), binary string=w304, byte order (0:big-endian, network order)=w289) -> (value=w292:u8)  [unwired: 2 in, 2 out]
              n92 = Unflatten From String(type=i64 0 ("default value 1"), binary string=w307, byte order (0:big-endian, network order)=w289) -> (value=w296:i64)  [unwired: 2 in, 2 out]
              n93 = Unflatten From String(type=0 ("default value 1"), binary string=w299, byte order (0:big-endian, network order)=w289) -> (value=w295:i32)  [unwired: 2 in, 2 out]
              n94 = Number To Boolean Array(number=w292) -> (Boolean array=w291:bool[])
              n95 = call "smartmeshIP to ni timestamp.vi"("use correction"=w288, "microeconds"=w295, "seconds"=w296) -> ("Dust Timestamp"=w294:timestamp)  [unwired: 8 in]
              n96 = case shown="46" w281 {
                tunnel: w294 -> [_ w348 w408]
                tunnel: w291 -> [_ w347 w407]
                tunnel: w289 -> [_ w338 w402]
                tunnel: [_ w327 w381] -> w286
                tunnel: w282 -> [_ w320 w394]
                frame 0, Default {
                }
                frame 46 {
                  n97 = String Subset(string=w320, offset (0)=14, length (rest)=4 ("length (rest)")) -> (substring=w358:string)
                  n98 = String Subset(string=w320, offset (0)=18, length (rest)=4 ("length (rest)")) -> (substring=w357:string)
                  n99 = String Subset(string=w320, offset (0)=26, length (rest)=2 ("length (rest)")) -> (substring=w354:string)
                  n100 = String Subset(string=w320, offset (0)=22, length (rest)=2 ("length (rest)")) -> (substring=w356:string)
                  n101 = String Subset(string=w320, offset (0)=32, length (rest)=2 ("length (rest)")) -> (substring=w350:string)
                  n102 = String Subset(string=w320, offset (0)=24, length (rest)=2 ("length (rest)")) -> (substring=w355:string)
                  n103 = String Subset(string=w320, offset (0)=28, length (rest)=2 ("length (rest)")) -> (substring=w353:string)
                  n104 = String Subset(string=w320, offset (0)=30, length (rest)=2 ("length (rest)")) -> (substring=w352:string)
                  n105 = String Subset(string=w320, offset (0)=36, length (rest)=2 ("length (rest)")) -> (substring=w343:string)
                  n106 = String Subset(string=w320, offset (0)=38, length (rest)=4 ("length (rest)")) -> (substring=w341:string)
                  n107 = String Subset(string=w320, offset (0)=42, length (rest)=4 ("length (rest)")) -> (substring=w339:string)
                  n108 = String Subset(string=w320, offset (0)=34, length (rest)=2 ("length (rest)")) -> (substring=w345:string)
                  n109 = Unflatten From String(type=sgl 0.0 ("default value 1"), binary string=w358, byte order (0:big-endian, network order)=w338) -> (value=w329:sgl)  [unwired: 2 in, 2 out]
                  n110 = Unflatten From String(type=u16 0 ("default value 1"), binary string=w355, byte order (0:big-endian, network order)=w338) -> (value=w314:u16)  [unwired: 2 in, 2 out]
                  n111 = Unflatten From String(type=u16 0 ("default value 1"), binary string=w356, byte order (0:big-endian, network order)=w338) -> (value=w312:u16)  [unwired: 2 in, 2 out]
                  n112 = Unflatten From String(type=u16 0 ("default value 1"), binary string=w354, byte order (0:big-endian, network order)=w338) -> (value=w313:u16)  [unwired: 2 in, 2 out]
                  n113 = Unflatten From String(type=u16 0 ("default value 1"), binary string=w353, byte order (0:big-endian, network order)=w338) -> (value=w315:u16)  [unwired: 2 in, 2 out]
                  n114 = Unflatten From String(type=sgl 0.0 ("default value 1"), binary string=w357, byte order (0:big-endian, network order)=w338) -> (value=w328:sgl)  [unwired: 2 in, 2 out]
                  n115 = Unflatten From String(type=u16 0 ("default value 1"), binary string=w352, byte order (0:big-endian, network order)=w338) -> (value=w323:u16)  [unwired: 2 in, 2 out]
                  n116 = Unflatten From String(type=u16 0 ("default value 1"), binary string=w350, byte order (0:big-endian, network order)=w338) -> (value=w324:u16)  [unwired: 2 in, 2 out]
                  n117 = Unflatten From String(type=u16 0 ("default value 1"), binary string=w343, byte order (0:big-endian, network order)=w338) -> (value=w326:u16)  [unwired: 2 in, 2 out]
                  n118 = Unflatten From String(type=sgl 0.0 ("default value 1"), binary string=w341, byte order (0:big-endian, network order)=w338) -> (value=w322:sgl)  [unwired: 2 in, 2 out]
                  n119 = Unflatten From String(type=sgl 0.0 ("default value 1"), binary string=w339, byte order (0:big-endian, network order)=w338) -> (value=w321:sgl)  [unwired: 2 in, 2 out]
                  n120 = Unflatten From String(type=u16 0 ("default value 1"), binary string=w345, byte order (0:big-endian, network order)=w338) -> (value=w325:u16)  [unwired: 2 in, 2 out]
                  n121 = To Long Integer(number=w314) -> (32bit integer=w318:i32)
                  n122 = To Long Integer(number=w315) -> (32bit integer=w316:i32)
                  n123 = To Long Integer(number=w313) -> (32bit integer=w317:i32)
                  n124 = To Long Integer(number=w312) -> (32bit integer=w319:i32)
                  n125 = Bundle("Dust Timestamp"=w348, "Boolean array"=w347, "default value 1"=w329, "default value 1"=w328, "default value 1"=w322, "default value 1"=w321, w319, w318, w317, w316, "default value 1"=w323, "default value 1"=w324, "default value 1"=w325, "default value 1"=w326) -> (w327:T27)  [unwired: 1 in]
                }
                frame 30 {
                  n126 = String Subset(string=w394, offset (0)=14, length (rest)=4 ("length (rest)")) -> (substring=w412:string)
                  n127 = String Subset(string=w394, offset (0)=20, length (rest)=2 ("length (rest)")) -> (substring=w410:string)
                  n128 = String Subset(string=w394, offset (0)=18, length (rest)=2 ("length (rest)")) -> (substring=w411:string)
                  n129 = String Subset(string=w394, offset (0)=22, length (rest)=2 ("length (rest)")) -> (substring=w409:string)
                  n130 = String Subset(string=w394, offset (0)=26, length (rest)=4 ("length (rest)")) -> (substring=w403:string)
                  n131 = String Subset(string=w394, offset (0)=24, length (rest)=2 ("length (rest)")) -> (substring=w405:string)
                  n132 = Unflatten From String(type=sgl 0.0 ("default value 1"), binary string=w412, byte order (0:big-endian, network order)=w402) -> (value=w397:sgl)  [unwired: 2 in, 2 out]
                  n133 = Unflatten From String(type=u16 0 ("default value 1"), binary string=w411, byte order (0:big-endian, network order)=w402) -> (value=w385:u16)  [unwired: 2 in, 2 out]
                  n134 = Unflatten From String(type=u16 0 ("default value 1"), binary string=w410, byte order (0:big-endian, network order)=w402) -> (value=w384:u16)  [unwired: 2 in, 2 out]
                  n135 = Unflatten From String(type=u16 0 ("default value 1"), binary string=w409, byte order (0:big-endian, network order)=w402) -> (value=w391:u16)  [unwired: 2 in, 2 out]
                  n136 = Unflatten From String(type=sgl 0.0 ("default value 1"), binary string=w403, byte order (0:big-endian, network order)=w402) -> (value=w395:sgl)  [unwired: 2 in, 2 out]
                  n137 = Unflatten From String(type=u16 0 ("default value 1"), binary string=w405, byte order (0:big-endian, network order)=w402) -> (value=w396:u16)  [unwired: 2 in, 2 out]
                  n138 = To Long Integer(number=w384) -> (32bit integer=w386:i32)
                  n139 = To Long Integer(number=w385) -> (32bit integer=w387:i32)
                  n140 = Bundle("Dust Timestamp"=w408, "Boolean array"=w407, "default value 1"=w397, "default value 1"=sgl 0.0, "default value 1"=w395, "default value 1"=sgl 0.0, w387, "default value 1"=0, w386, "default value 1"=0, "default value 1"=w391, "default value 1"=u16 0, "default value 1"=w396, "default value 1"=u16 0) -> (w381:T28)  [unwired: 1 in]
                }
              }
              n141 = Unbundle(w285) -> (w284:bool)  [unwired: 2 out]
              n142 = case shown="False" w284 {
                tunnel: w285 -> [w428 w432]
                tunnel: [w425 w429] -> w283
                frame False {
                  n143 = Get Date/Time In Seconds() -> (seconds since 1Jan1904=w424:timestamp)
                  n144 = Bundle(cluster=w428, TRUE, "default value 1"=u16 1, "seconds since 1Jan1904"=w424) -> (w425:T14)
                }
                frame True {
                  n145 = Unbundle(w432) -> ("default value 1"=w430:u16)  [unwired: 2 out]
                  n146 = Increment(x=w430) -> (x+1=w431:u16)
                  n147 = Bundle(cluster=w432, "default value 1"=w431) -> (w429:T14)  [unwired: 2 in]
                }
              }
            }
            frame 9 {
              w441 = T18."little-endian" ("byte order (0:big-endian, network order)")
              # "differential avalanch packets  - singned int16"
              n148 = String Length(string=w434) -> (length=w433:i32)
              n149 = String Subset(string=w434, offset (0)=1, length (rest)=8 ("length (rest)")) -> (substring=w459:string)
              n150 = String Subset(string=w434, offset (0)=13, length (rest)=1 ("length (rest)")) -> (substring=w456:string)
              n151 = String Subset(string=w434, offset (0)=9, length (rest)=4 ("length (rest)")) -> (substring=w451:string)
              n152 = Unflatten From String(type=u8 0 ("default value 1"), binary string=w456, byte order (0:big-endian, network order)=w441) -> (value=w444:u8)  [unwired: 2 in, 2 out]
              n153 = Unflatten From String(type=i64 0 ("default value 1"), binary string=w459, byte order (0:big-endian, network order)=w441) -> (value=w448:i64)  [unwired: 2 in, 2 out]
              n154 = Unflatten From String(type=0 ("default value 1"), binary string=w451, byte order (0:big-endian, network order)=w441) -> (value=w447:i32)  [unwired: 2 in, 2 out]
              n155 = Number To Boolean Array(number=w444) -> (Boolean array=w443:bool[])
              n156 = call "smartmeshIP to ni timestamp.vi"("use correction"=w440, "microeconds"=w447, "seconds"=w448) -> ("Dust Timestamp"=w446:timestamp)  [unwired: 8 in]
              n157 = case shown="30" w433 {
                tunnel: w446 -> [_ w500 w560]
                tunnel: w443 -> [_ w499 w559]
                tunnel: w441 -> [_ w490 w554]
                tunnel: [_ w479 w533] -> w438
                tunnel: w434 -> [_ w472 w546]
                frame 0, Default {
                }
                frame 46 {
                  n158 = String Subset(string=w472, offset (0)=14, length (rest)=4 ("length (rest)")) -> (substring=w510:string)
                  n159 = String Subset(string=w472, offset (0)=18, length (rest)=4 ("length (rest)")) -> (substring=w509:string)
                  n160 = String Subset(string=w472, offset (0)=26, length (rest)=2 ("length (rest)")) -> (substring=w506:string)
                  n161 = String Subset(string=w472, offset (0)=22, length (rest)=2 ("length (rest)")) -> (substring=w508:string)
                  n162 = String Subset(string=w472, offset (0)=32, length (rest)=2 ("length (rest)")) -> (substring=w502:string)
                  n163 = String Subset(string=w472, offset (0)=24, length (rest)=2 ("length (rest)")) -> (substring=w507:string)
                  n164 = String Subset(string=w472, offset (0)=28, length (rest)=2 ("length (rest)")) -> (substring=w505:string)
                  n165 = String Subset(string=w472, offset (0)=30, length (rest)=2 ("length (rest)")) -> (substring=w504:string)
                  n166 = String Subset(string=w472, offset (0)=36, length (rest)=2 ("length (rest)")) -> (substring=w495:string)
                  n167 = String Subset(string=w472, offset (0)=38, length (rest)=4 ("length (rest)")) -> (substring=w493:string)
                  n168 = String Subset(string=w472, offset (0)=42, length (rest)=4 ("length (rest)")) -> (substring=w491:string)
                  n169 = String Subset(string=w472, offset (0)=34, length (rest)=2 ("length (rest)")) -> (substring=w497:string)
                  n170 = Unflatten From String(type=sgl 0.0 ("default value 1"), binary string=w510, byte order (0:big-endian, network order)=w490) -> (value=w481:sgl)  [unwired: 2 in, 2 out]
                  n171 = Unflatten From String(type=i16 0 ("default value 1"), binary string=w507, byte order (0:big-endian, network order)=w490) -> (value=w466:i16)  [unwired: 2 in, 2 out]
                  n172 = Unflatten From String(type=i16 0 ("default value 1"), binary string=w508, byte order (0:big-endian, network order)=w490) -> (value=w464:i16)  [unwired: 2 in, 2 out]
                  n173 = Unflatten From String(type=i16 0 ("default value 1"), binary string=w506, byte order (0:big-endian, network order)=w490) -> (value=w465:i16)  [unwired: 2 in, 2 out]
                  n174 = Unflatten From String(type=i16 0 ("default value 1"), binary string=w505, byte order (0:big-endian, network order)=w490) -> (value=w467:i16)  [unwired: 2 in, 2 out]
                  n175 = Unflatten From String(type=sgl 0.0 ("default value 1"), binary string=w509, byte order (0:big-endian, network order)=w490) -> (value=w480:sgl)  [unwired: 2 in, 2 out]
                  n176 = Unflatten From String(type=u16 0 ("default value 1"), binary string=w504, byte order (0:big-endian, network order)=w490) -> (value=w475:u16)  [unwired: 2 in, 2 out]
                  n177 = Unflatten From String(type=u16 0 ("default value 1"), binary string=w502, byte order (0:big-endian, network order)=w490) -> (value=w476:u16)  [unwired: 2 in, 2 out]
                  n178 = Unflatten From String(type=u16 0 ("default value 1"), binary string=w495, byte order (0:big-endian, network order)=w490) -> (value=w478:u16)  [unwired: 2 in, 2 out]
                  n179 = Unflatten From String(type=sgl 0.0 ("default value 1"), binary string=w493, byte order (0:big-endian, network order)=w490) -> (value=w474:sgl)  [unwired: 2 in, 2 out]
                  n180 = Unflatten From String(type=sgl 0.0 ("default value 1"), binary string=w491, byte order (0:big-endian, network order)=w490) -> (value=w473:sgl)  [unwired: 2 in, 2 out]
                  n181 = Unflatten From String(type=u16 0 ("default value 1"), binary string=w497, byte order (0:big-endian, network order)=w490) -> (value=w477:u16)  [unwired: 2 in, 2 out]
                  n182 = To Long Integer(number=w466) -> (32bit integer=w470:i32)
                  n183 = To Long Integer(number=w467) -> (32bit integer=w468:i32)
                  n184 = To Long Integer(number=w465) -> (32bit integer=w469:i32)
                  n185 = To Long Integer(number=w464) -> (32bit integer=w471:i32)
                  n186 = Bundle("Dust Timestamp"=w500, "Boolean array"=w499, "default value 1"=w481, "default value 1"=w480, "default value 1"=w474, "default value 1"=w473, w471, w470, w469, w468, "default value 1"=w475, "default value 1"=w476, "default value 1"=w477, "default value 1"=w478) -> (w479:T27)  [unwired: 1 in]
                }
                frame 30 {
                  n187 = String Subset(string=w546, offset (0)=14, length (rest)=4 ("length (rest)")) -> (substring=w564:string)
                  n188 = String Subset(string=w546, offset (0)=20, length (rest)=2 ("length (rest)")) -> (substring=w562:string)
                  n189 = String Subset(string=w546, offset (0)=18, length (rest)=2 ("length (rest)")) -> (substring=w563:string)
                  n190 = String Subset(string=w546, offset (0)=22, length (rest)=2 ("length (rest)")) -> (substring=w561:string)
                  n191 = String Subset(string=w546, offset (0)=26, length (rest)=4 ("length (rest)")) -> (substring=w555:string)
                  n192 = String Subset(string=w546, offset (0)=24, length (rest)=2 ("length (rest)")) -> (substring=w557:string)
                  n193 = Unflatten From String(type=sgl 0.0 ("default value 1"), binary string=w564, byte order (0:big-endian, network order)=w554) -> (value=w549:sgl)  [unwired: 2 in, 2 out]
                  n194 = Unflatten From String(type=i16 0 ("default value 1"), binary string=w563, byte order (0:big-endian, network order)=w554) -> (value=w537:i16)  [unwired: 2 in, 2 out]
                  n195 = Unflatten From String(type=i16 0 ("default value 1"), binary string=w562, byte order (0:big-endian, network order)=w554) -> (value=w536:i16)  [unwired: 2 in, 2 out]
                  n196 = Unflatten From String(type=u16 0 ("default value 1"), binary string=w561, byte order (0:big-endian, network order)=w554) -> (value=w543:u16)  [unwired: 2 in, 2 out]
                  n197 = Unflatten From String(type=sgl 0.0 ("default value 1"), binary string=w555, byte order (0:big-endian, network order)=w554) -> (value=w547:sgl)  [unwired: 2 in, 2 out]
                  n198 = Unflatten From String(type=u16 0 ("default value 1"), binary string=w557, byte order (0:big-endian, network order)=w554) -> (value=w548:u16)  [unwired: 2 in, 2 out]
                  n199 = To Long Integer(number=w536) -> (32bit integer=w538:i32)
                  n200 = To Long Integer(number=w537) -> (32bit integer=w539:i32)
                  n201 = Bundle("Dust Timestamp"=w560, "Boolean array"=w559, "default value 1"=w549, "default value 1"=sgl 0.0, "default value 1"=w547, "default value 1"=sgl 0.0, w539, "default value 1"=0, w538, "default value 1"=0, "default value 1"=w543, "default value 1"=u16 0, "default value 1"=w548, "default value 1"=u16 0) -> (w533:T28)  [unwired: 1 in]
                }
              }
              n202 = Unbundle(w437) -> (w436:bool)  [unwired: 2 out]
              n203 = case shown="False" w436 {
                tunnel: w437 -> [w580 w584]
                tunnel: [w577 w581] -> w435
                frame False {
                  n204 = Get Date/Time In Seconds() -> (seconds since 1Jan1904=w576:timestamp)
                  n205 = Bundle(cluster=w580, TRUE, "default value 1"=u16 1, "seconds since 1Jan1904"=w576) -> (w577:T14)
                }
                frame True {
                  n206 = Unbundle(w584) -> ("default value 1"=w582:u16)  [unwired: 2 out]
                  n207 = Increment(x=w582) -> (x+1=w583:u16)
                  n208 = Bundle(cluster=w584, "default value 1"=w583) -> (w581:T14)  [unwired: 2 in]
                }
              }
            }
            frame 2 {
              (unwired) u16 0
              n209 = Bundle(cluster=w591, TRUE, "default value 1"=u16 0, "seconds since 1Jan1904"=w585) -> (w590:T14)
            }
            frame 3 {
              w601 = T18."little-endian" ("byte order (0:big-endian, network order)")
              n210 = String Length(string=w597) -> (length=w603:i32)
              n211 = Greater?(x=w603, y=5) -> (0:w616:bool)
              n212 = Greater?(x=w603, y=17) -> (0:w600:bool)
              n213 = Unbundle(w621) -> ("default value 1"=w608:u16, "seconds since 1Jan1904"=w618:timestamp)  [unwired: 1 out]
              n214 = case shown="True" w616 {
                tunnel: w601 -> [_ w659]
                tunnel: w597 -> [_ w658]
                tunnel: [w654 w655] -> w606
                tunnel: w618 -> [w654 _]
                tunnel: w604 -> [_ w656]
                frame False {
                }
                frame True {
                  n215 = String Subset(string=w658, offset (0)=3, length (rest)=8 ("length (rest)")) -> (substring=w666:string)
                  n216 = String Subset(string=w658, offset (0)=11, length (rest)=4 ("length (rest)")) -> (substring=w663:string)
                  n217 = Unflatten From String(type=i64 0 ("default value 1"), binary string=w666, byte order (0:big-endian, network order)=w659) -> (value=w661:i64)  [unwired: 2 in, 2 out]
                  n218 = Unflatten From String(type=0 ("default value 1"), binary string=w663, byte order (0:big-endian, network order)=w659) -> (value=w660:i32)  [unwired: 2 in, 2 out]
                  n219 = call "smartmeshIP to ni timestamp.vi"("use correction"=w656, "microeconds"=w660, "seconds"=w661) -> ("Dust Timestamp"=w655:timestamp)  [unwired: 8 in]
                }
              }
              n220 = case shown="True" w600 {
                tunnel: w601 -> [_ w635]
                tunnel: w597 -> [_ w636]
                tunnel: [u16 0 ("default value 1") w643] -> w599
                tunnel: [213.5 w634] -> w598
                frame False {
                }
                frame True {
                  n221 = String Subset(string=w636, offset (0)=17, length (rest)=2 ("length (rest)")) -> (substring=w645:string)
                  n222 = String Subset(string=w636, offset (0)=15, length (rest)=2 ("length (rest)")) -> (substring=w640:string)
                  n223 = Unflatten From String(type=u16 0 ("default value 1"), binary string=w645, byte order (0:big-endian, network order)=w635) -> (value=w643:u16)  [unwired: 2 in, 2 out]
                  "num_samples" <- w643
                  n224 = Unflatten From String(type=u16 0 ("default value 1"), binary string=w640, byte order (0:big-endian, network order)=w635) -> (value=w638:u16)  [unwired: 2 in, 2 out]
                  n225 = Divide(x=w638, y=u16 100) -> (x/y=w634:dbl)
                  "sps" <- w634
                  "data" <- w636
                }
              }
              n226 = String Subset(string=w597, offset (0)=1, length (rest)=2 ("length (rest)")) -> (substring=w626:string)
              n227 = Unflatten From String(type=u16 0 ("default value 1"), binary string=w626, byte order (0:big-endian, network order)=w601) -> (value=w612:u16)  [unwired: 2 in, 2 out]
              n228 = Bundle("default value 1"=w612, "Dust Timestamp"=w606, "default value 1"=w608, w598, "default value 1"=w599) -> (w619:T29)  [unwired: 1 in]
              n229 = Less Or Equal?(x=w608, y=u16 0) -> (x <= y?=w609:bool)
              n230 = Bundle(cluster=w621, FALSE) -> (w623:T14)  [unwired: 2 in]
              n231 = And(x="list only event > 0", y=w609) -> (x .and. y?=w614:bool)
              n232 = case shown="False" w614 {
                tunnel: [w651 w653] -> w624
                tunnel: w620 -> [w650 w653]
                tunnel: w619 -> [w649 _]
                tunnel: w611 -> [w648 _]
                tunnel: [w648 u8 100] -> w610
                frame False {
                  n233 = Build Array (concatenate)(w649, w650) -> (w651:T30)
                }
                frame True {
                }
              }
            }
            frame 4 {
              w680 = u32 1 ("y")
              w677 = T18."little-endian" ("byte order (0:big-endian, network order)")
              n234 = String Length(string=w673) -> (length=w672:i32)
              n235 = Greater?(x=w672, y=57) -> (0:w670:bool)
              n236 = case shown="False" w670 {
                tunnel: w673 -> [w765 w777]
                tunnel: w677 -> [w764 w776]
                tunnel: [w763 w775] -> w676
                tunnel: [w762 w774] -> w675
                frame False {
                  n237 = String Subset(string=w765, offset (0)=56, length (rest)=1 ("length (rest)")) -> (substring=w766:string)
                  n238 = String Subset(string=w765, offset (0)=55, length (rest)=1 ("length (rest)")) -> (substring=w767:string)
                  n239 = Unflatten From String(type=u8 0 ("default value 1"), binary string=w766, byte order (0:big-endian, network order)=w764) -> (value=w762:u8)  [unwired: 2 in, 2 out]
                  n240 = Unflatten From String(type=u8 0 ("default value 1"), binary string=w767, byte order (0:big-endian, network order)=w764) -> (value=w763:u8)  [unwired: 2 in, 2 out]
                }
                frame True {
                  n241 = String Subset(string=w777, offset (0)=57, length (rest)=2 ("length (rest)")) -> (substring=w778:string)
                  n242 = String Subset(string=w777, offset (0)=55, length (rest)=2 ("length (rest)")) -> (substring=w779:string)
                  n243 = Unflatten From String(type=u16 0 ("default value 1"), binary string=w778, byte order (0:big-endian, network order)=w776) -> (value=w774:u16)  [unwired: 2 in, 2 out]
                  n244 = Unflatten From String(type=u16 0 ("default value 1"), binary string=w779, byte order (0:big-endian, network order)=w776) -> (value=w775:u16)  [unwired: 2 in, 2 out]
                }
              }
              n245 = String Subset(string=w673, offset (0)=1, length (rest)=4 ("length (rest)")) -> (substring=w729:string)
              n246 = String Subset(string=w673, offset (0)=5, length (rest)=4 ("length (rest)")) -> (substring=w712:string)
              n247 = String Subset(string=w673, offset (0)=9, length (rest)=4 ("length (rest)")) -> (substring=w711:string)
              n248 = String Subset(string=w673, offset (0)=17, length (rest)=4 ("length (rest)")) -> (substring=w709:string)
              n249 = String Subset(string=w673, offset (0)=13, length (rest)=4 ("length (rest)")) -> (substring=w710:string)
              n250 = String Subset(string=w673, offset (0)=21, length (rest)=4 ("length (rest)")) -> (substring=w708:string)
              n251 = String Subset(string=w673, offset (0)=33, length (rest)=4 ("length (rest)")) -> (substring=w705:string)
              n252 = String Subset(string=w673, offset (0)=25, length (rest)=4 ("length (rest)")) -> (substring=w707:string)
              n253 = String Subset(string=w673, offset (0)=45, length (rest)=4 ("length (rest)")) -> (substring=w702:string)
              n254 = String Subset(string=w673, offset (0)=29, length (rest)=4 ("length (rest)")) -> (substring=w706:string)
              n255 = String Subset(string=w673, offset (0)=37, length (rest)=4 ("length (rest)")) -> (substring=w704:string)
              n256 = String Subset(string=w673, offset (0)=41, length (rest)=4 ("length (rest)")) -> (substring=w703:string)
              n257 = String Subset(string=w673, offset (0)=49, length (rest)=4 ("length (rest)")) -> (substring=w701:string)
              n258 = String Subset(string=w673, offset (0)=54, length (rest)=1 ("length (rest)")) -> (substring=w688:string)
              n259 = String Subset(string=w673, offset (0)=53, length (rest)=1 ("length (rest)")) -> (substring=w689:string)
              n260 = Unflatten From String(type=u32 0 ("default value 1"), binary string=w711, byte order (0:big-endian, network order)=w677) -> (value=w699:u32)  [unwired: 2 in, 2 out]
              n261 = Unflatten From String(type=u32 0 ("default value 1"), binary string=w712, byte order (0:big-endian, network order)=w677) -> (value=w700:u32)  [unwired: 2 in, 2 out]
              n262 = Unflatten From String(type=sgl 0.0 ("default value 1"), binary string=w710, byte order (0:big-endian, network order)=w677) -> (value=w698:sgl)  [unwired: 2 in, 2 out]
              n263 = Unflatten From String(type=sgl 0.0 ("default value 1"), binary string=w709, byte order (0:big-endian, network order)=w677) -> (value=w697:sgl)  [unwired: 2 in, 2 out]
              n264 = Unflatten From String(type=sgl 0.0 ("default value 1"), binary string=w708, byte order (0:big-endian, network order)=w677) -> (value=w696:sgl)  [unwired: 2 in, 2 out]
              n265 = Unflatten From String(type=u32 0 ("default value 1"), binary string=w729, byte order (0:big-endian, network order)=w677) -> (value=w727:u32)  [unwired: 2 in, 2 out]
              n266 = Unflatten From String(type=sgl 0.0 ("default value 1"), binary string=w706, byte order (0:big-endian, network order)=w677) -> (value=w694:sgl)  [unwired: 2 in, 2 out]
              n267 = Unflatten From String(type=sgl 0.0 ("default value 1"), binary string=w707, byte order (0:big-endian, network order)=w677) -> (value=w695:sgl)  [unwired: 2 in, 2 out]
              n268 = Unflatten From String(type=sgl 0.0 ("default value 1"), binary string=w705, byte order (0:big-endian, network order)=w677) -> (value=w693:sgl)  [unwired: 2 in, 2 out]
              n269 = Unflatten From String(type=sgl 0.0 ("default value 1"), binary string=w704, byte order (0:big-endian, network order)=w677) -> (value=w692:sgl)  [unwired: 2 in, 2 out]
              n270 = Unflatten From String(type=sgl 0.0 ("default value 1"), binary string=w703, byte order (0:big-endian, network order)=w677) -> (value=w691:sgl)  [unwired: 2 in, 2 out]
              n271 = Unflatten From String(type=u32 0 ("default value 1"), binary string=w702, byte order (0:big-endian, network order)=w677) -> (value=w681:u32)  [unwired: 2 in, 2 out]
              n272 = Unflatten From String(type=u32 0 ("default value 1"), binary string=w701, byte order (0:big-endian, network order)=w677) -> (value=w682:u32)  [unwired: 2 in, 2 out]
              n273 = Unflatten From String(type=u8 0 ("default value 1"), binary string=w688, byte order (0:big-endian, network order)=w677) -> (value=w687:u8)  [unwired: 2 in, 2 out]
              n274 = Unflatten From String(type=u8 0 ("default value 1"), binary string=w689, byte order (0:big-endian, network order)=w677) -> (value=w690:u8)  [unwired: 2 in, 2 out]
              n275 = Multiply(x=w681, y=w680) -> (x*y=w679:u32)
              n276 = Multiply(x=w682, y=w680) -> (x*y=w678:u32)
              n277 = Bundle("default value 1"=w727, "default value 1"=w700, "default value 1"=w699, "default value 1"=w698, "default value 1"=w697, "default value 1"=w696, "default value 1"=w695, "default value 1"=w694, "default value 1"=w693, "default value 1"=w692, "default value 1"=w691, w679, w678, "default value 1"=w690, "default value 1"=w687, "default value 1"=w676, "default value 1"=w675) -> (w730:T31)  [unwired: 1 in]
            }
            frame 5 {
              w799 = T18."little-endian" ("byte order (0:big-endian, network order)")
              n278 = String Subset(string=w800, offset (0)=5, length (rest)=2 ("length (rest)")) -> (substring=w824:string)
              n279 = String Subset(string=w800, offset (0)=1, length (rest)=2 ("length (rest)")) -> (substring=w827:string)
              n280 = String Subset(string=w800, offset (0)=3, length (rest)=2 ("length (rest)")) -> (substring=w820:string)
              n281 = String Subset(string=w800, offset (0)=7, length (rest)=2 ("length (rest)")) -> (substring=w813:string)
              n282 = String Subset(string=w800, offset (0)=9, length (rest)=8 ("length (rest)")) -> (substring=w809:string)
              n283 = String Subset(string=w800, offset (0)=17, length (rest)=4 ("length (rest)")) -> (substring=w807:string)
              n284 = String Subset(string=w800, offset (0)=21, length (rest)=1 ("length (rest)")) -> (substring=w802:string)
              n285 = Unflatten From String(type=u16 0 ("default value 1"), binary string=w824, byte order (0:big-endian, network order)=w799) -> ()  [unwired: 2 in, 3 out]
              n286 = Unflatten From String(type=u16 0 ("default value 1"), binary string=w827, byte order (0:big-endian, network order)=w799) -> (value=w789:u16)  [unwired: 2 in, 2 out]
              n287 = Unflatten From String(type=u16 0 ("default value 1"), binary string=w820, byte order (0:big-endian, network order)=w799) -> ()  [unwired: 2 in, 3 out]
              n288 = Unflatten From String(type=u16 0 ("default value 1"), binary string=w813, byte order (0:big-endian, network order)=w799) -> ()  [unwired: 2 in, 3 out]
              n289 = Unflatten From String(type=i64 0 ("default value 1"), binary string=w809, byte order (0:big-endian, network order)=w799) -> (value=w795:i64)  [unwired: 2 in, 2 out]
              n290 = Unflatten From String(type=0 ("default value 1"), binary string=w807, byte order (0:big-endian, network order)=w799) -> (value=w796:i32)  [unwired: 2 in, 2 out]
              n291 = Unflatten From String(type=u8 0 ("default value 1"), binary string=w802, byte order (0:big-endian, network order)=w799) -> ()  [unwired: 2 in, 3 out]
              n292 = call "smartmeshIP to ni timestamp.vi"("use correction"=w787, "microeconds"=w796, "seconds"=w795) -> ("Dust Timestamp"=w790:timestamp)  [unwired: 8 in]
              n293 = Bundle(cluster=T17 {"ID"=0, "Timestamp"=timestamp(0 s since 1904-01-01), "Num"=0, "Rødt lys"=427.0, "Num 2"=0}, "ID"=w789, "Timestamp"=w790) -> (w791:T17)  [unwired: 3 in]
              n294 = Build Array (concatenate)(w791, w794) -> (w793:T30)
            }
            frame 6 {
              w850 = T18."little-endian" ("byte order (0:big-endian, network order)")
              # "Downloaded data single ended - uint16"
              n295 = String Length(string=w846) -> (length=w849:i32)
              n296 = String Subset(string=w846, offset (0)=4, length (rest)=4 ("length (rest)")) -> (substring=w865:string)
              n297 = String Subset(string=w846, offset (0)=1, length (rest)=2 ("length (rest)")) -> (substring=w868:string)
              n298 = String Subset(string=w846, offset (0)=3, length (rest)=1 ("length (rest)")) -> (substring=w861:string)
              n299 = String Subset(string=w846, offset (0)=8, length (rest)=4 ("length (rest)")) -> (substring=w853:string)
              n300 = Subtract(x=w849, y=12 ("length")) -> (x-y=w848:i32)
              n301 = Unflatten From String(type=u32 0 ("default value 1"), binary string=w865, byte order (0:big-endian, network order)=w850) -> (value=w837:u32)  [unwired: 2 in, 2 out]
              n302 = Unflatten From String(type=u16 0 ("default value 1"), binary string=w868, byte order (0:big-endian, network order)=w850) -> (value=w859:u16)  [unwired: 2 in, 2 out]
              n303 = Unflatten From String(type=u8 0 ("default value 1"), binary string=w861, byte order (0:big-endian, network order)=w850) -> (value=w836:u8)  [unwired: 2 in, 2 out]
              n304 = Unflatten From String(type=u32 0 ("default value 1"), binary string=w853, byte order (0:big-endian, network order)=w850) -> (value=w851:u32)  [unwired: 2 in, 2 out]
              n305 = Number To Boolean Array(number=w836) -> (Boolean array=w839:bool[])
              n306 = Boolean To (0,1)(Boolean=w839) -> (0, 1=w838:i16[])
              n307 = Add Array Elements(numeric array=w838) -> (sum=w835:i16)
              n308 = Multiply(x=w835, y=i16 2) -> (x*y=w833:i16)
              n309 = Divide(x=w848, y=w833) -> (x/y=w847:dbl)
              n310 = for {
                N: w847 -> [_]
                shift-right: [w875] -> _
                shift-left: u32 12 -> [w876]
                tunnel: w846 -> [w877]
                tunnel: [w874] -> w841 mode=indexing
                tunnel: w835 -> [w873]
                n311 = for {
                  N: w873 -> [_]
                  shift-right: [w882] -> w875
                  shift-left: w876 -> [w881]
                  tunnel: w877 -> [w885]
                  tunnel: [w878] -> w874 mode=indexing
                  n312 = Increment(x=w881) -> (x+1=w883:u32)
                  n313 = String Subset(string=w885, offset (0)=w881, length (rest)=2 ("length (rest)")) -> (substring=w886:string)
                  n314 = Increment(x=w883) -> (x+1=w882:u32)
                  n315 = Unflatten From String(type=u16 0 ("default value 1"), binary string=w886, byte order (0:big-endian, network order)=T18."little-endian") -> (value=w879:u16)  [unwired: 2 in, 2 out]
                  n316 = To Long Integer(number=w879) -> (32bit integer=w878:i32)
                }
              }
              n317 = Bundle("default value 1"=w859, "default value 1"=w836, "default value 1"=w837, "default value 1"=w851, w841) -> (w842:T15)  [unwired: 1 in]
            }
            frame 10 {
              w906 = T18."little-endian" ("byte order (0:big-endian, network order)")
              # "Downloaded data differential - int16"
              n318 = String Length(string=w902) -> (length=w905:i32)
              n319 = String Subset(string=w902, offset (0)=4, length (rest)=4 ("length (rest)")) -> (substring=w921:string)
              n320 = String Subset(string=w902, offset (0)=1, length (rest)=2 ("length (rest)")) -> (substring=w924:string)
              n321 = String Subset(string=w902, offset (0)=3, length (rest)=1 ("length (rest)")) -> (substring=w917:string)
              n322 = String Subset(string=w902, offset (0)=8, length (rest)=4 ("length (rest)")) -> (substring=w909:string)
              n323 = Subtract(x=w905, y=12 ("length")) -> (x-y=w904:i32)
              n324 = Unflatten From String(type=u32 0 ("default value 1"), binary string=w921, byte order (0:big-endian, network order)=w906) -> (value=w893:u32)  [unwired: 2 in, 2 out]
              n325 = Unflatten From String(type=u16 0 ("default value 1"), binary string=w924, byte order (0:big-endian, network order)=w906) -> (value=w915:u16)  [unwired: 2 in, 2 out]
              n326 = Unflatten From String(type=u8 0 ("default value 1"), binary string=w917, byte order (0:big-endian, network order)=w906) -> (value=w892:u8)  [unwired: 2 in, 2 out]
              n327 = Unflatten From String(type=u32 0 ("default value 1"), binary string=w909, byte order (0:big-endian, network order)=w906) -> (value=w907:u32)  [unwired: 2 in, 2 out]
              n328 = Number To Boolean Array(number=w892) -> (Boolean array=w895:bool[])
              n329 = Boolean To (0,1)(Boolean=w895) -> (0, 1=w894:i16[])
              n330 = Add Array Elements(numeric array=w894) -> (sum=w891:i16)
              n331 = Multiply(x=w891, y=i16 2) -> (x*y=w889:i16)
              n332 = Divide(x=w904, y=w889) -> (x/y=w903:dbl)
              n333 = for {
                N: w903 -> [_]
                shift-right: [w931] -> _
                shift-left: u32 12 -> [w932]
                tunnel: w902 -> [w933]
                tunnel: [w930] -> w897 mode=indexing
                tunnel: w891 -> [w929]
                n334 = for {
                  N: w929 -> [_]
                  shift-right: [w938] -> w931
                  shift-left: w932 -> [w937]
                  tunnel: w933 -> [w941]
                  tunnel: [w935] -> w930 mode=indexing
                  n335 = Increment(x=w937) -> (x+1=w939:u32)
                  n336 = String Subset(string=w941, offset (0)=w937, length (rest)=2 ("length (rest)")) -> (substring=w942:string)
                  n337 = Increment(x=w939) -> (x+1=w938:u32)
                  n338 = Unflatten From String(type=i16 0 ("default value 1"), binary string=w942, byte order (0:big-endian, network order)=T18."little-endian") -> (value=w934:i16)  [unwired: 2 in, 2 out]
                  n339 = To Long Integer(number=w934) -> (32bit integer=w935:i32)
                }
              }
              n340 = Bundle("default value 1"=w915, "default value 1"=w892, "default value 1"=w893, "default value 1"=w907, w897) -> (w898:T15)  [unwired: 1 in]
            }
            frame 7 {
              w950 = u8 4 ("length")
              w951 = u8 0 ("index")
              w974 = T18."little-endian" ("byte order (0:big-endian, network order)")
              # "OMSG_AUX data packet"
              n341 = String Length(string=w948) -> (length=w947:i32)
              n342 = Greater?(x=w947, y=8 ("offset (0)")) -> (0:w945:bool)
              n343 = case shown="True" w945 {
                tunnel: w974 -> [_ w1032]
                tunnel: [_ w1026] -> w953
                tunnel: [_ w1025] -> w952
                tunnel: w948 -> [_ w1024]
                frame False {
                }
                frame True {
                  w1033 = 9 ("y")
                  n344 = String Length(string=w1024) -> (length=w1037:i32)
                  n345 = Subtract(x=w1037, y=w1033) -> (x-y=w1035:i32)
                  n346 = String Subset(string=w1024, offset (0)=8, length (rest)=1 ("length (rest)")) -> (substring=w1028:string)
                  n347 = Divide(x=w1035, y=2.0) -> (x/y=w1034:dbl)
                  n348 = Unflatten From String(type=u8 0 ("default value 1"), binary string=w1028) -> (value=w1027:u8)  [unwired: 3 in, 2 out]
                  n349 = Number To Boolean Array(number=w1027) -> (Boolean array=w1025:bool[])
                  n350 = for {
                    N: w1034 -> [_]
                    tunnel: w1024 -> [w1048]
                    tunnel: w1032 -> [w1040]
                    tunnel: w1033 -> [w1044]
                    tunnel: [w1042] -> w1026 mode=indexing
                    tunnel: w1025 -> [w1041] mode=indexing
                    i -> [w1043]
                    n351 = Multiply(x=w1043, y=2) -> (x*y=w1050:i32)
                    n352 = Add(x=w1050, y=w1044) -> (x+y=w1049:i32)
                    n353 = String Subset(string=w1048, offset (0)=w1049, length (rest)=2 ("length (rest)")) -> (substring=w1039:string)
                    n354 = case shown="False" w1041 {
                      tunnel: w1040 -> [w1056 w1061]
                      tunnel: w1039 -> [w1055 w1062]
                      tunnel: [w1053 w1058] -> w1038
                      frame False {
                        n355 = Unflatten From String(type=u16 0 ("default value 1"), binary string=w1055, byte order (0:big-endian, network order)=w1056) -> (value=w1054:u16)  [unwired: 2 in, 2 out]
                        n356 = To Double Precision Float(number=w1054) -> (double precision float=w1053:dbl)
                      }
                      frame True {
                        n357 = Unflatten From String(type=i16 0 ("default value 1"), binary string=w1062, byte order (0:big-endian, network order)=w1061) -> (value=w1059:i16)  [unwired: 2 in, 2 out]
                        n358 = To Double Precision Float(number=w1059) -> (double precision float=w1058:dbl)
                      }
                    }
                    n359 = Divide(x=2.5 ("dt"), y=65535.0 ("dt")) -> (x/y=w1045:dbl)
                    n360 = Multiply(x=w1038, y=w1045) -> (x*y=w1042:dbl)
                  }
                }
              }
              n361 = String Subset(string=w948, offset (0)=3, length (rest)=1 ("length (rest)")) -> (substring=w1016:string)
              n362 = String Subset(string=w948, offset (0)=1, length (rest)=1 ("length (rest)")) -> (substring=w1019:string)
              n363 = String Subset(string=w948, offset (0)=2, length (rest)=1 ("length (rest)")) -> (substring=w1012:string)
              n364 = String Subset(string=w948, offset (0)=4, length (rest)=2 ("length (rest)")) -> (substring=w985:string)
              n365 = String Subset(string=w948, offset (0)=6, length (rest)=2 ("length (rest)")) -> (substring=w979:string)
              n366 = Unflatten From String(type=u8 0 ("default value 1"), binary string=w1016, byte order (0:big-endian, network order)=w974) -> (value=w994:u8)  [unwired: 2 in, 2 out]
              n367 = Unflatten From String(type=u8 0 ("default value 1"), binary string=w1019, byte order (0:big-endian, network order)=w974) -> (value=w971:u8)  [unwired: 2 in, 2 out]
              n368 = Unflatten From String(type=u8 0 ("default value 1"), binary string=w1012, byte order (0:big-endian, network order)=w974) -> (value=w970:u8)  [unwired: 2 in, 2 out]
              n369 = Unflatten From String(type=u16 0 ("default value 1"), binary string=w985, byte order (0:big-endian, network order)=w974) -> (value=w983:u16)  [unwired: 2 in, 2 out]
              n370 = Unflatten From String(type=i16 0 ("default value 1"), binary string=w979, byte order (0:big-endian, network order)=w974) -> (value=w977:i16)  [unwired: 2 in, 2 out]
              n371 = Number To Boolean Array(number=w994) -> (Boolean array=w972:bool[])
              n372 = Number To Boolean Array(number=w970) -> (Boolean array=w968:bool[])
              n373 = Number To Boolean Array(number=w971) -> (Boolean array=w969:bool[])
              n374 = Divide(x=2.5 ("dt"), y=65535.0 ("dt")) -> (x/y=w991:dbl)
              n375 = Divide(x=w977, y=100.0 ("dt")) -> (x/y=w949:dbl)
              n376 = Multiply(x=w983, y=w991) -> (x*y=w982:dbl)
              n377 = Array Subset(array=w969, index=w950, length=w950) -> (w967:bool[])
              n378 = Array Subset(array=w969, index=w951, length=w950) -> (w966:bool[])
              n379 = Array Subset(array=w968, index=w950, length=w950) -> (w965:bool[])
              n380 = Array Subset(array=w968, index=w951, length=w950) -> (w964:bool[])
              n381 = Boolean Array To Number(Boolean array=w965) -> (number=w961:u32)
              n382 = Boolean Array To Number(Boolean array=w966) -> (number=w960:u32)
              n383 = Boolean Array To Number(Boolean array=w967) -> (number=w963:u32)
              n384 = Boolean Array To Number(Boolean array=w964) -> (number=w962:u32)
              n385 = To Unsigned Byte Integer(number=w961) -> (unsigned 8bit integer=w957:u8)
              n386 = To Unsigned Byte Integer(number=w960) -> (unsigned 8bit integer=w958:u8)
              n387 = To Unsigned Byte Integer(number=w963) -> (unsigned 8bit integer=w959:u8)
              n388 = To Unsigned Byte Integer(number=w962) -> (unsigned 8bit integer=w956:u8)
              n389 = Get Date/Time In Seconds() -> (seconds since 1Jan1904=w1001:timestamp)
              n390 = Bundle(w959, w958, w957, w956) -> (w955:cluster{u8, u8, u8, u8})  [unwired: 1 in]
              n391 = Get Date/Time In Seconds() -> (seconds since 1Jan1904=w997:timestamp)
              n392 = Build Array(w949) -> (w1005:dbl[])
              n393 = Bundle By Name("Y"=w1005, "t0"=w1001) -> (w1004:waveform(dbl))  [unwired: 1 in]
              n394 = Multiply(x=3.0, y=w982) -> (x*y=w989:dbl)
              n395 = Add(x=0.69, y=w989) -> (x+y=w981:dbl)
              n396 = Build Array(w981) -> (w1000:dbl[])
              n397 = Bundle By Name("Y"=w1000, "t0"=w997) -> (w999:waveform(dbl))  [unwired: 1 in]
              n398 = Bundle(w955, "Boolean array"=w972, w981, w949, "Boolean array"=w952, w953, "seconds since 1Jan1904"=w954) -> (w975:T32)  [unwired: 1 in]
              n399 = Set Waveform Attribute(5:w996, 6:"NI_ChannelName" ("name"), 7:w999) -> (3:w995:waveform(dbl))  [unwired: 1 in, 2 out]
              n400 = Set Waveform Attribute(5:w996, 6:"NI_ChannelName" ("name"), 7:w1004) -> (3:w1002:waveform(dbl))  [unwired: 1 in, 2 out]
            }
            frame 100, Default {
            }
          }
        }
      }
    }
    n401 = Unbundle By Name(w61) -> ("MAC Adress"=w66:string, "data"=w65:string)  [unwired: 3 out]
    n402 = String Length(string=w65) -> (length=w68:i32)
    n403 = Greater Than 0?(x=w68) -> (x > 0?=w67:bool)
    n404 = case shown="True" w67 {
      tunnel: w66 -> [_ w1098]
      tunnel: w65 -> [_ w1097]
      tunnel: [w1093 w1095] -> w64
      tunnel: w63 -> [w1093 w1094]
      frame False {
      }
      frame True {
        n405 = Bundle("MAC Adress"=w1098, "data"=w1097) -> (w1096:cluster{"MAC Adress":string, "data":string})  [unwired: 1 in]
        n406 = Build Array (concatenate)(w1096, w1094) -> (w1095:cluster{"MAc Adress":string, "data":string}[])
      }
    }
  }
  "NGI  packets dust" <- w23
  "last packet type" <- w21
  "Avalanch Packets" <- w19
  "Is Logging" <- w17
  "Downloaded dataset" <- w16
  "Adjustable Parameters" <- w12
  "AUX data" <- w8
  "Avalanch JBV" <- w2
  n407 = Transpose 2D Array(2D array=w14) -> (transposed array=→"Recent events":T33)
  n408 = Bundle(w6, w5) -> (→"output waveforms":cluster{waveform(dbl)[], waveform(dbl)[]})  [unwired: 1 in]
